vi "wheeltrackerGo_Stop8.6.vi"() -> ()   [LabVIEW 2013]
uses:
  pass_fail.ctl
  <vilib>/DAQmx/write.llb/DAQmx Write (Digital Bool 1Line 1Point).vi
  <vilib>/DAQmx/read.llb/DAQmx Read (Analog DBL 1Chan 1Samp).vi
  <vilib>/DAQmx/read.llb/DAQmx Read (Digital Bool 1Line 1Point).vi
  <vilib>/DAQmx/create/channels.llb/DAQmx Create Channel (DO-Digital Output).vi
  <vilib>/DAQmx/miscellaneous.llb/DAQmx Fill In Error Info.vi
  <vilib>/DAQmx/create/channels.llb/DAQmx Create Channel (DI-Digital Input).vi
  <vilib>/DAQmx/create/channels.llb/DAQmx Create Channel (AI-Voltage-Basic).vi
  <vilib>/Utility/file.llb/Write To Spreadsheet File (string).vi
  <vilib>/Utility/file.llb/Write To Spreadsheet File (DBL).vi
panel:
  out "Sample Time Interval (ms)":u32=20
  in  "Sample Rate (Hz)":u32=50 min=1 max=200
  out "Elapsed Time (s)":dbl
  out "x-y 2":dbl
  out "Time has Elapsed":bool
  in  "Time Before Delay End":dbl
  in  "Camera Trigger":tag="Dev2/port0/line3"
  in  "Lick Thr":dbl
  out "Ana Lick?":bool
  in  "x":dbl=1.0
  out "x*y":dbl
  in  "Scale":dbl=1.0 format="%#_13g"
  in  "Analog Lick Chan":tag="Dev2/ai0"
  out "Prev Stim?":bool
  in  "Alternate Stim?":bool
  in  "Thr Opto \nRun Factor":dbl=0.05
  out "Opto RUN Thr":bool
  in  "Opto Channel":tag="Dev2/port0/line4"
  in  "Opto Cond":T1(radio)=enum."Opto OFF"
  out "OptoON":bool
  in  "min speed":dbl=0.005
  in  "Stop Before Go?":bool
  in  "Fails 2 Penalty":dbl=3.0
  in  "Fails Penalty (s)":dbl=4.0
  out "Conseq. Fails":i32
  in  "control puff interval":dbl=1.0
  in  "control puff":bool
  in  "lick fail":bool
  out "NoGo & Stop":bool caption="Boolean"
  in  "NoGo Prob?":dbl
  out "NoGo?":bool
  in  "No-Go/Stop Channel":tag="Dev2/port0/line6"
  out "Success %":dbl
  in  "Buffer Time (s)":dbl
  in  "Stop Fail Repeat Prob 2":dbl caption="STOP\nRepeat Prob on fail"
  out "In":bool
  in  "Digital In Channel":tag="Dev2/port0/line5"
  out "Stop Speed Reached":bool
  out "Go/Stop?":bool
  out "Stop Flash # 2":dbl
  in  "Stop Stim On (s)":dbl=0.5 format="%#_13g"
  out "Stop Delay \nActual (s)":dbl
  in  "Delay Max (s)":dbl=4.0 format="%#_13g"
  in  "Delay Min (s)":dbl=2.0 format="%#_13g"
  out "Stop Thres Reached":bool
  in  "Stop Thres.":dbl=1.0 format="%#_13g"
  in  "Stop Flash #":dbl
  in  "Stim On (s)":dbl=0.1 format="%#_13g"
  out "Speed":dbl format="%#_13g"
  in  "Stop":bool
  in  "Stop Fail Speed":dbl=3.0
  out "Stop Slide":dbl(slide) max=2.0 scale=0.0..2.0
  in  "Stop Prob":dbl=0.5 caption="Probability" min=0.0 max=1.0 step=0.1 format="%.1f"
  in  "Stop Duration":dbl=2.0 caption="Stop Dur (s)"
  in  "Current Period":u8
  in  "Current Trial":u16
  in  "Fail sound play":bool
  in  "Pass sound play":bool
  in  "Fail Sound":string(combo)="C:\\Windows\\Media\\ringout.wav"
  in  "Pass Sound":string(combo)="C:\\Windows\\Media\\windows error.wav"
  in  "Fail Repeat Prob":dbl caption="GO\nRepeat Prob on fail"
  out "reset distance":bool
  out "give reward":bool
  in  "Shutter Click":bool
  out "Slide Trial #":u8(slide) max=5 scale=0.0..5.0
  out "Current Thres":dbl
  in  "exit":bool
  in  "Go/noGo Reward Thres":dbl=5.0 caption="Threshold"
  in  "Wheel Test":bool
  in  "Init Abort Threshold":dbl=6.0 caption="Abort Threshold"
  in  "Room light test":bool
  in  "Solid test":bool
  in  "Flash test":bool
  out "Go/No-go LED":bool
  in  "Room Light Channel":tag="Dev2/port0/line0"
  in  "Shutter Duration":dbl=0.05
  in  "Wheel Monitor Channel":refnum<visa-resource-name>="USB0::0x046D::0xC245::NI-VISA-0::RAW"
  in  "Number of Trials":u16=1
  out "Room light":bool
  out "Slide Inter-trail":dbl(slide) max=6.0 scale=-1.0..6.0
  out "Fail Delay Actual":dbl caption="Actual(s)"
  in  "Fail Delay Max":dbl=6.0 caption="Max(s)"
  in  "Fail Delay Min":dbl=6.0 caption="Min(s)"
  out "Pass Delay Actual":dbl caption="Actual(s)"
  in  "Pass Delay Max":dbl=3.0 caption="Max(s)"
  in  "Pass delay Min":dbl=3.0 caption="Min(s)"
  in  "Reward time (s)":dbl=2.0
  out "Slide Reward":dbl(slide) max=2.0 scale=0.0..2.0
  out "Slide go/no-go":dbl(slide) max=12.0 scale=0.0..12.0
  out "Slide Delay":dbl(slide) max=18.879 scale=0.0..18.879
  out "Thres reached":bool
  in  "Go Duration":dbl=12.0 caption="Go Dur (s)"
  out "Init Delay Actual":dbl caption="Actual(s)"
  in  "Init Delay Max":dbl=2.0 caption="Max(s)"
  in  "Init Delay Min(s)":dbl=1.0 caption="Min(s)"
  in  "Flashing Interval":dbl=0.1
  in  "Go Channel":tag="Dev2/port0/line1"
  in  "Data File Location":path
  in  "Queue":T2
  in  "Save":bool=TRUE
  in  "Log rate":dbl=0.01 min=0.0 max=1.0
  in  "Lin rate":dbl=0.01 min=0.0 max=1.0
  in  "Exp rate":dbl=0.01 min=0.0 max=1.0
  in  "Decay":enum32{"None", "Exp", "Lin", "Log"}(radio)
  in  "Wheel direction":bool=TRUE
  out "Shutter":bool
  in  "Run Trials":bool
  in  "Shutter Channel":tag="Dev2/port0/line2"
  out "Distance":dbl
  out "Reward Count":dbl
  out "Wheel Graph":cluster{dbl, dbl, i16, dbl, dbl}(graph)
  # "NOT USED"
  # "Initial Delay Period"
  # "Go/No-Go Period"
  # "Stop Period"
  # "Reward Period"
  # "Inter-trial Delay Period"
  # "Go-Stop Delay"
  # "Pass"
  # "Fail"
  # "*Update data saving parameters*"
  # "Decay rate"
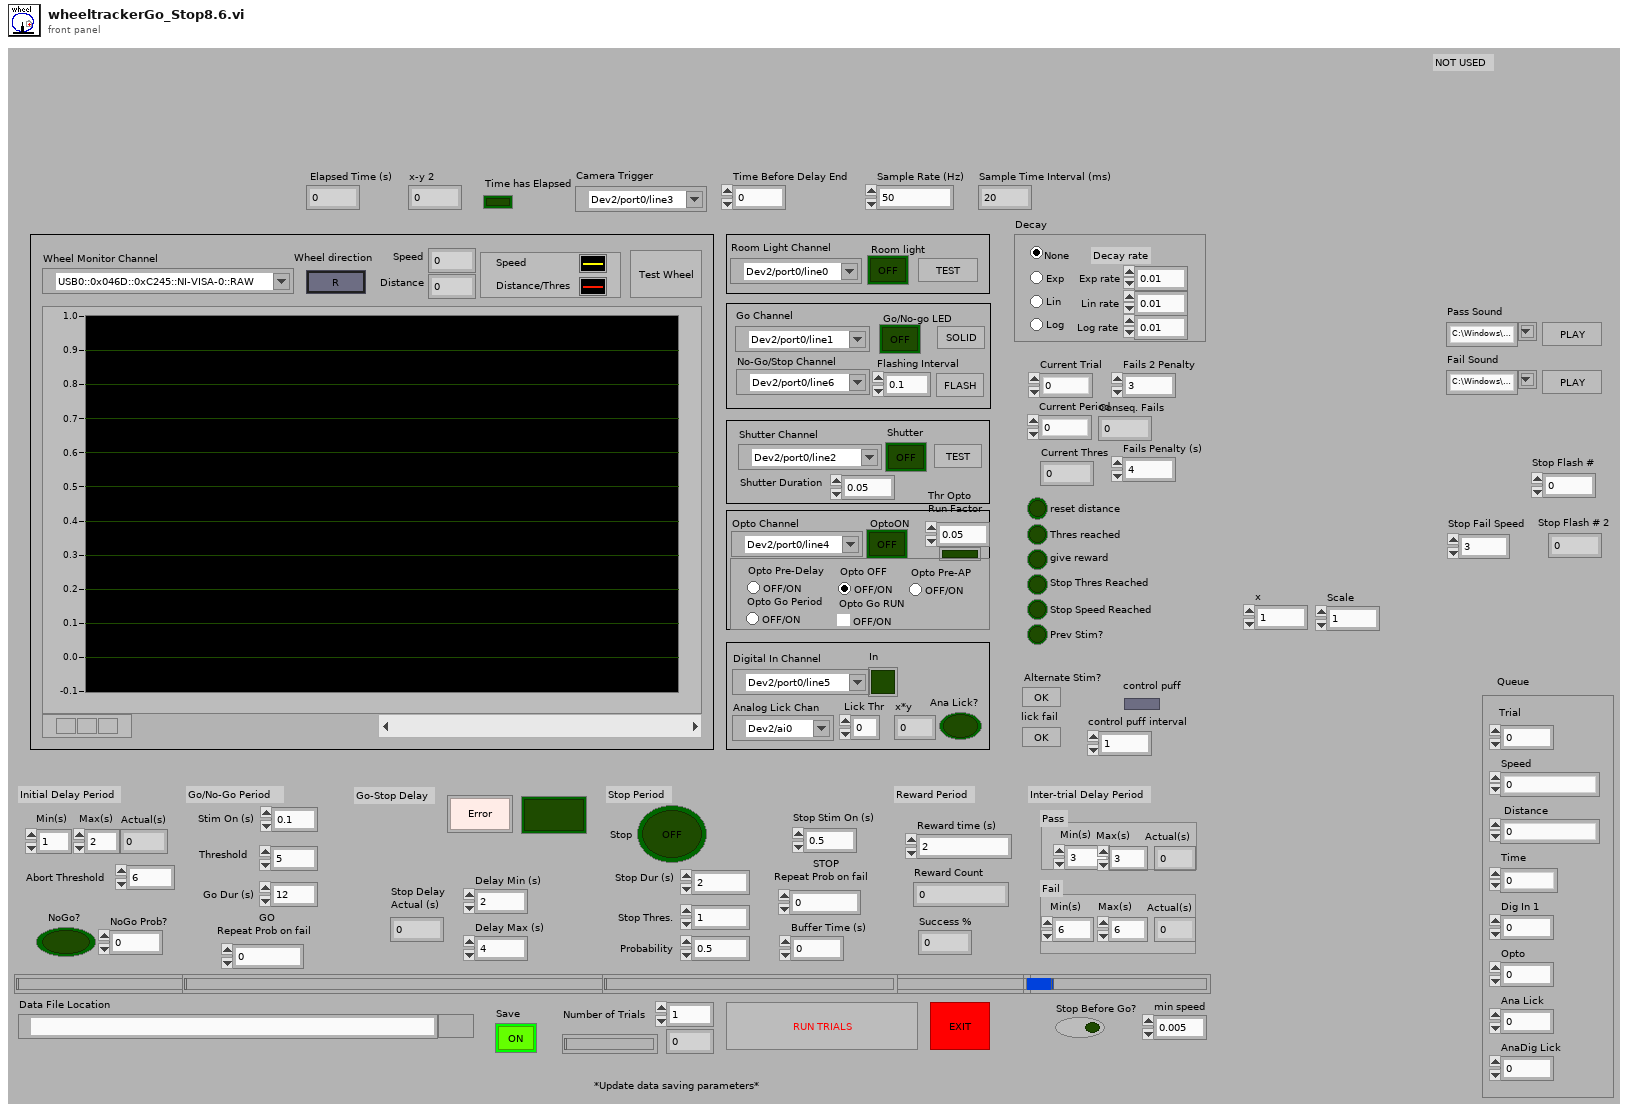
[diagram p1: front panel]
types:
  T1 = enum32{"Opto Pre-Delay", "Opto Go Period", "Opto OFF", "Opto Go RUN", "Opto Pre-AP"}
  T2 = cluster{"Trial":dbl, "Speed":dbl, " Distance":dbl, "Time":dbl, "Dig In 1":dbl, "Opto":dbl, "Ana Lick":dbl, "AnaDig Lick":dbl}
  T3 = enum16{"open", "replace", "create", "open or create", "replace or create", "replace or create with confirmation"}
  T4 = typedef "pass_fail.ctl" = enum32{"passed", "init fail", "go/no-go fail", "Stop Fail", "aborted"}
  T5 = cluster{"task out":refnum<k21>, "task out":refnum<k21>}
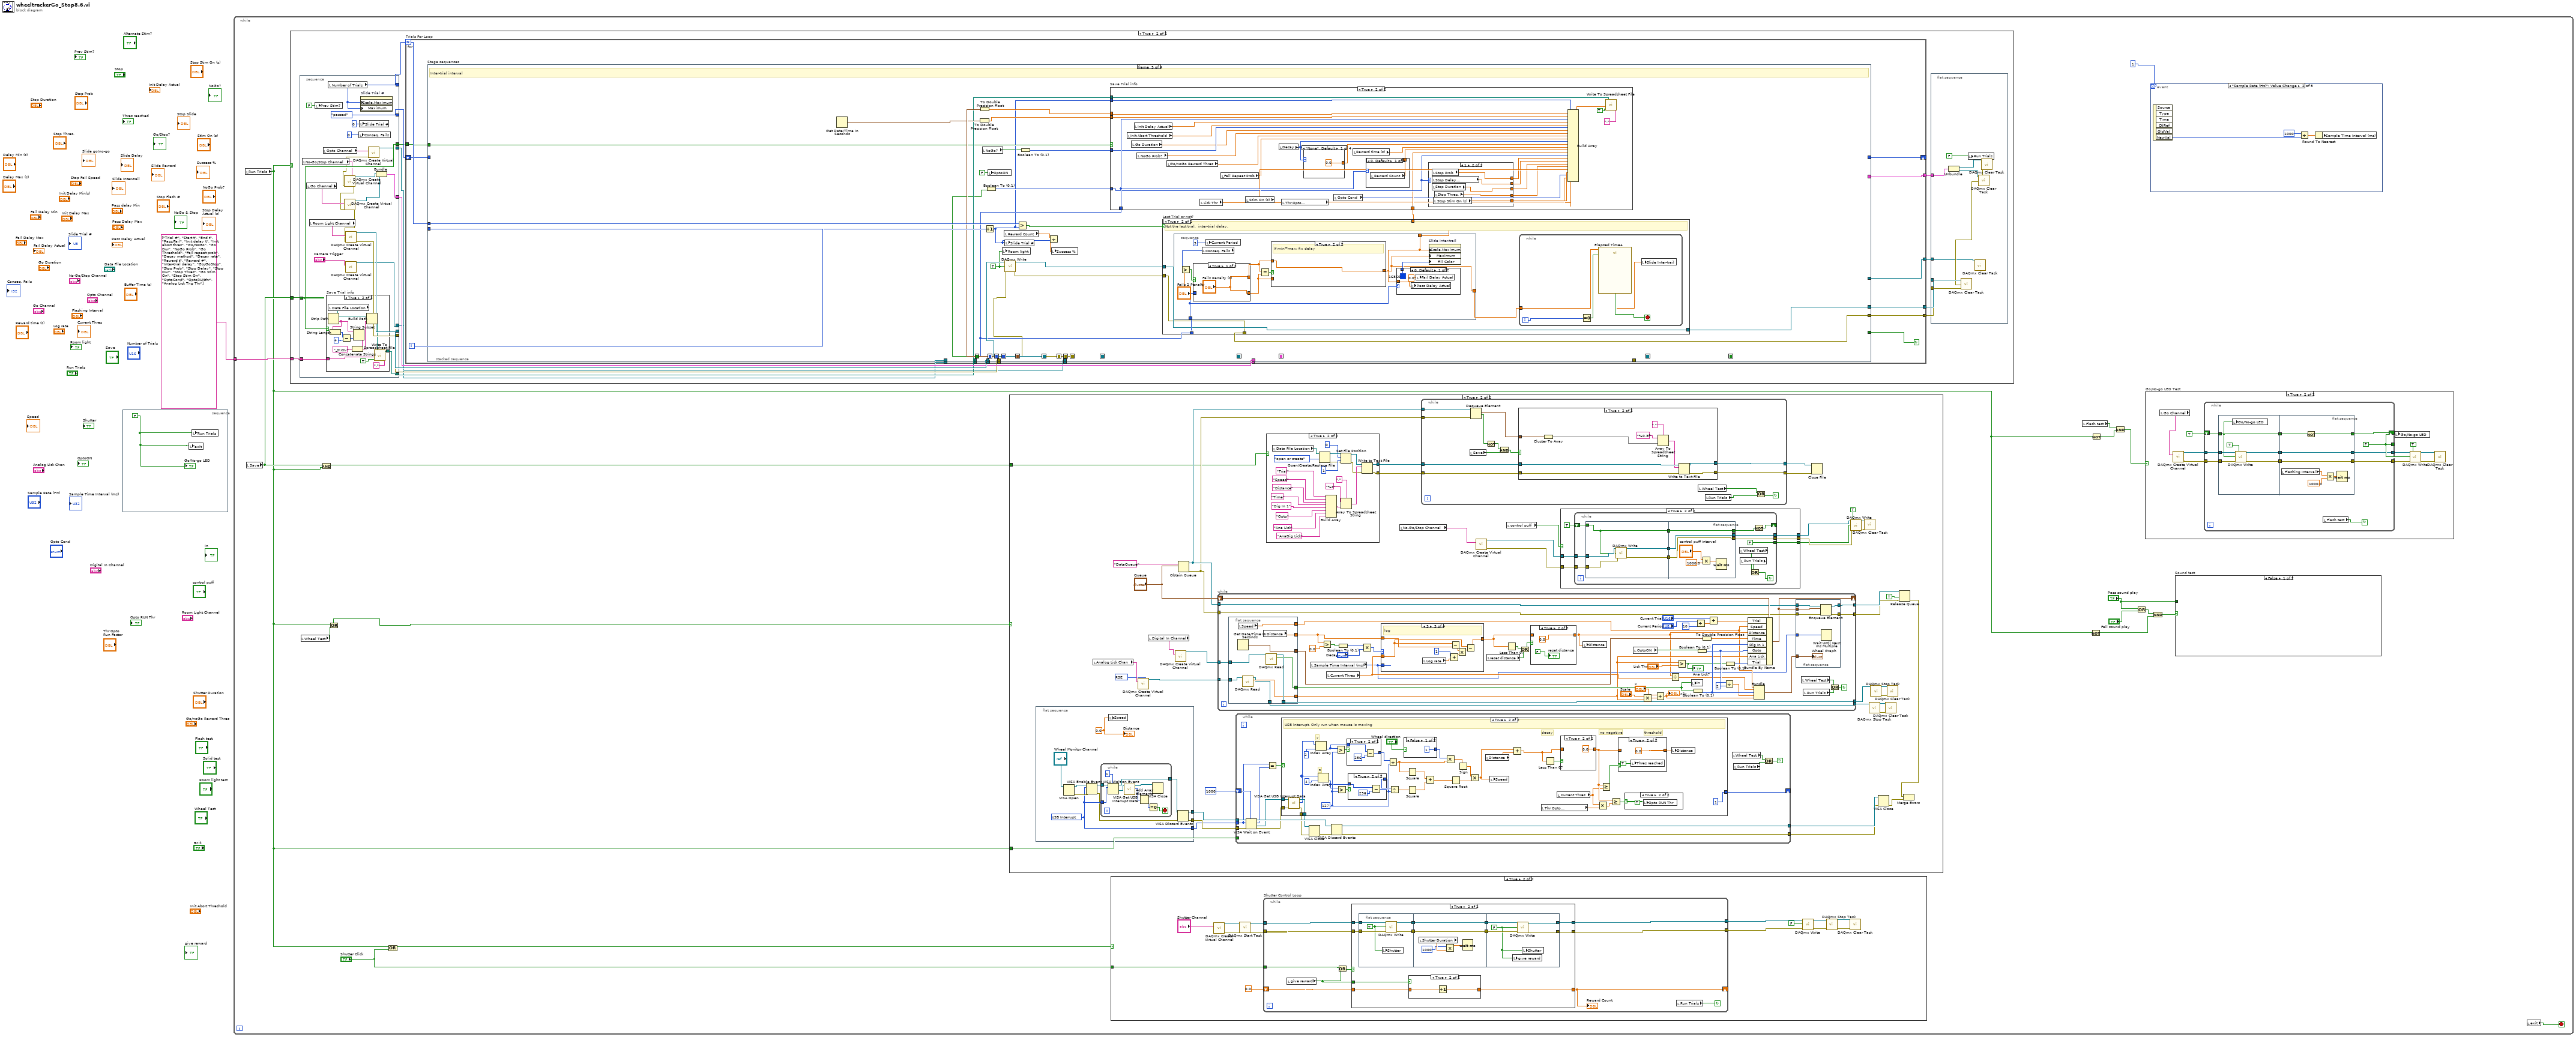
[diagram p0: block diagram]
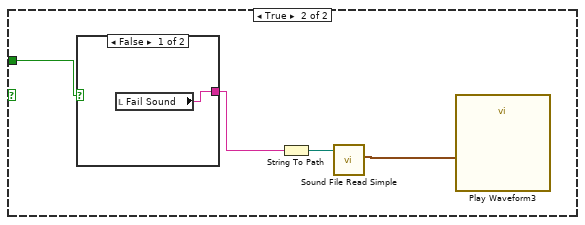
[diagram p3: hidden frame]
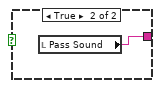
[diagram p4: hidden frame]
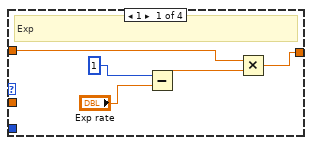
[diagram p10: hidden frame]
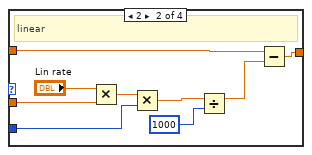
[diagram p11: hidden frame]
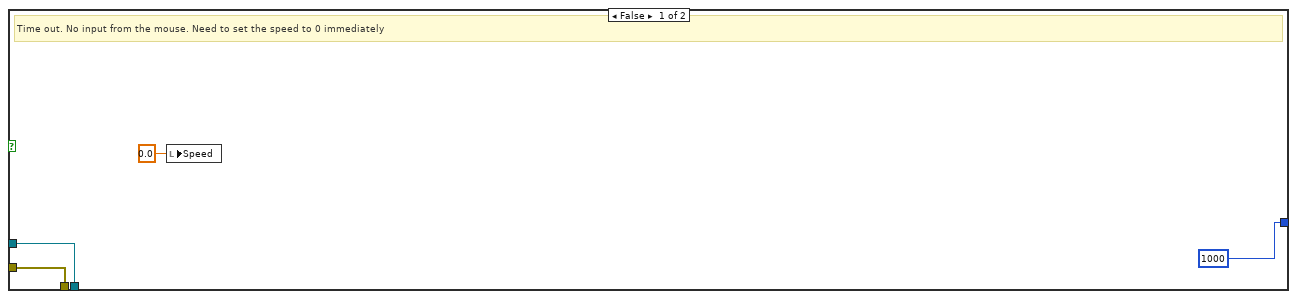
[diagram p13: hidden frame]
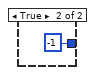
[diagram p17: hidden frame]
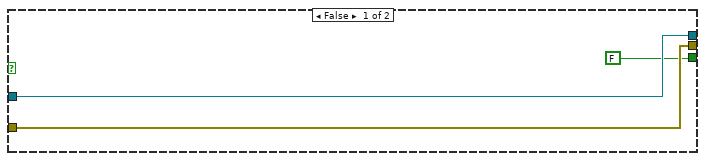
[diagram p20: hidden frame]
diagram:
  n1 = stacked-sequence {
    frame #0 {
      w2 = FALSE ("start")
      n2 = local write "exit"(w2) -> ()
      n3 = local write "Run Trials"(w2) -> ()
      "Go/No-go LED" <- w2
    }
  }
  n4 = while {
    tunnel: string[] ["Trial #", "Start t", "End t", "Pass/Fail", "Init delay t", "Init abort thres", "Go/NoGo", "Go Dur", "NoGo Prob", "Go Threshold", "Fail repeat prob", "Decay method", "Decay rate", "Reward t", "Reward #", "Inter-trial delay", "Go/GoStop", "Stop Prob", "Stop Delay", "Stop Dur", "Stop Thres", "Go Stim On", "Stop Stim On", "OptoCond", "OptoRUNthr", "Analog Lick Trig Thr"] -> [w8]
    stop <- w20 stop-if-true
    n5 = local read "Run Trials"() -> (w5:bool)
    n6 = local read "Save"() -> (w7:bool)
    n7 = case shown="True" w5 {
      tunnel: w8 -> [_ w464]
      tunnel: w7 -> [_ w463]
      frame False {
      }
      frame True {
        n8 = stacked-sequence {
          tunnel: [w505] -> w473
          tunnel: [w502] -> w472
          tunnel: [w490] -> w471
          tunnel: [w500] -> w468
          tunnel: [pass_fail."passed" ("How it ended")] -> w466
          tunnel: [w498] -> w465
          tunnel: w464 -> [w497]
          tunnel: w463 -> [w496]
          tunnel: [w496] -> w462
          tunnel: [w487] -> w461
          tunnel: [w483] -> w460
          frame #0 {
            n9 = local read "No-Go/Stop Channel"() -> (w493:tag)
            n10 = local read "Go Channel"() -> (w495:tag)
            n11 = local read "Room Light Channel"() -> (w503:tag)
            n12 = local write "Prev Stim?"(FALSE ("Prev Stim?")) -> ()
            n13 = local read "Opto Channel"() -> (w488:tag)
            n14 = case "Save Trial info" shown="True" w496 {
              tunnel: [_ w509] -> w498
              tunnel: w497 -> [_ w508]
              frame False {
              }
              frame True {
                n15 = local read "Data File Location"() -> (w519:path)
                n16 = Strip Path(path=w519) -> (stripped path=w512:path, name=w518:string)
                n17 = String Length(string=w518) -> (length=w516:i32)
                n18 = Subtract(x=w516, y=4) -> (x-y=w510:i32)
                n19 = String Subset(string=w518, length (rest)=w510) -> (substring=w515:string)  [unwired: 1 in]
                n20 = Concatenate Strings(w515, "_tr.csv") -> (w513:string)
                n21 = Build Path(base path=w512, name or relative path=w513) -> (appended path=w511:path)
                n22 = call-poly <vilib>:"Write To Spreadsheet File.vi"("delimiter (\\t)"="," ("delimiter (\\t)"), "append to file? (new file:F)"=TRUE, "1D data"=w508, "file path (dialog if empty)"=w511) -> ("new file path (Not A Path if cancelled)"=w509:path)  [unwired: 4 in]
              }
            }
            n23 = local read "Number of Trials"() -> (w505:u16)
            n24 = call-poly <vilib>:"DAQmx Create Virtual Channel.vi"("lines"="Camera Trigger") -> ("task out"=w483:refnum<k21>)  [unwired: 13 in, 1 out]
            n25 = local write "Conseq. Fails"(u8 0 ("Slide Trial #")) -> ()
            n26 = local write "Slide Trial #"(u8 0 ("Slide Trial #")) -> ()
            n27 = property on="Slide Trial #" class="Slide (strict)"("Scale.Maximum"=w505, "Maximum"=w505) -> ()  [unwired: 2 in, 2 out]
            n28 = call-poly <vilib>:"DAQmx Create Virtual Channel.vi"("lines"=w488) -> ("task out"=w487:refnum<k21>, "error out"=w486:errorcluster)  [unwired: 13 in]
            n29 = call-poly <vilib>:"DAQmx Create Virtual Channel.vi"("lines"=w493, "error in"=w486) -> ("task out"=w491:refnum<k21>, "error out"=w494:errorcluster)  [unwired: 12 in]
            n30 = call-poly <vilib>:"DAQmx Create Virtual Channel.vi"("lines"=w495, "error in"=w494) -> ("task out"=w492:refnum<k21>, "error out"=w501:errorcluster)  [unwired: 12 in]
            n31 = call-poly <vilib>:"DAQmx Create Virtual Channel.vi"("lines"=w503, "error in"=w501) -> ("task out"=w502:refnum<k21>, "error out"=w500:errorcluster)  [unwired: 12 in]
            n32 = Bundle("task out"=w491, "task out"=w492) -> (w490:T5)  [unwired: 1 in]
          }
        }
        n33 = for "Trials For Loop" {
          N: w473 -> [w534]
          tunnel: w472 -> [w533]
          tunnel: w471 -> [w532]
          tunnel: [w523] -> w470
          tunnel: [w531] -> w469
          tunnel: w468 -> [w530]
          tunnel: [w529] -> w467
          shift-right: [w526] -> _
          shift-left: w466 -> [w527]
          tunnel: w465 -> [w525]
          tunnel: w462 -> [w524]
          tunnel: w461 -> [w522]
          tunnel: w460 -> [w521]
          tunnel: [w520] -> w459
          i -> [w535]
          stop <- w528 continue-if-true
          # "Repeat Trials  For loop."
          n34 = stacked-sequence "Stage sequences" {
            seq-local: [w563 _ _ _ _ _] -> [_ w678 _ _ _ _]
            seq-local: [_ _ w858 _ _ _] -> [_ _ _ w920 w957 _]
            seq-local: [w561 _ _ _ _ _] -> [_ _ _ _ w965 _]
            seq-local: [w549 _ _ _ _ _] -> [_ w676 _ _ _ _]
            seq-local: [_ w675 _ _ _ _] -> [_ _ w857 _ _ _]
            seq-local: [w550 _ _ _ _ _] -> [_ _ _ _ w963 _]
            seq-local: [_ w673 _ _ _ _] -> [_ _ w852 _ _ _]
            seq-local: [_ w671 _ _ _ _] -> [_ _ w853 _ _ _]
            seq-local: [_ _ w856 _ _ _] -> [_ _ _ _ w955 _]
            seq-local: [_ w672 _ _ _ _] -> [_ _ w854 _ _ _]
            seq-local: [_ _ w852 _ _ _] -> [_ _ _ _ w950 _]
            seq-local: [w548 _ _ _ _ _] -> [_ w670 _ _ _ _]
            seq-local: [_ w669 _ _ _ _] -> [_ _ _ _ _ _]
            seq-local: [w538 _ _ _ _ _] -> [_ _ w851 _ _ _]
            tunnel: w535 -> [w546 w668 _ _ w968 _]
            tunnel: w534 -> [_ _ _ _ w967 _]
            tunnel: w533 -> [w562 _ _ _ _ _]
            tunnel: w532 -> [_ w677 _ _ _ _]
            tunnel: [_ _ _ _ w953 _] -> w531
            tunnel: w530 -> [w560 _ _ _ _ _]
            tunnel: [_ _ _ _ w951 _] -> w529
            tunnel: [_ _ _ _ _ w1068] -> w528
            tunnel: w527 -> [_ w674 _ _ _ _]
            tunnel: [_ _ _ w920 _ _] -> w526
            tunnel: w525 -> [_ _ _ _ w959 _]
            tunnel: w524 -> [_ _ _ _ w956 _]
            tunnel: [_ _ w855 _ _ _] -> w523
            tunnel: w522 -> [w555 _ _ _ _ _]
            tunnel: w521 -> [w545 _ _ _ _ _]
            tunnel: [w536 _ _ _ _ _] -> _
            tunnel: [_ _ w851 _ _ _] -> w520
            frame #0 {
              w547 = FALSE ("data")
              # "Fix/Random Initial Delay"
              n35 = flat-sequence {
                tunnel: w562 -> [w587]
                tunnel: [w586] -> w561
                tunnel: w560 -> [w585]
                tunnel: [w584] -> w551
                tunnel: [w581] -> w550
                tunnel: w546 -> [w580]
                tunnel: [w588] -> w559
                tunnel: [w603] -> w564
                tunnel: w559 -> [w603]
                frame #0 {
                  w574 = FALSE
                  w583 = FALSE ("data")
                  w577 = 0.0
                  n36 = Increment(x=w580) -> (x+1=w579:i32)
                  n37 = Get Date/Time In Seconds() -> (seconds since 1Jan1904=w581:timestamp)
                  n38 = local write "Current Trial"(w579) -> ()
                  n39 = local write "Current Period"(1) -> ()
                  n40 = local write "Stop Thres Reached"(w574) -> ()
                  n41 = local write "Thres reached"(w574) -> ()
                  n42 = local write "reset distance"(TRUE) -> ()
                  n43 = local write "give reward"(w574) -> ()
                  n44 = local write "OptoON"(w574) -> ()
                  n45 = local read "Init Delay Min(s)"() -> (w575:dbl)
                  n46 = local read "Init Delay Max"() -> (w582:dbl)
                  n47 = local write "Room light"(w583) -> ()
                  n48 = call-poly <vilib>:"DAQmx Write.vi"("task/channels in"=w587, "data"=w583, "error in"=w585) -> ("task out"=w586:refnum<k21>, "error out"=w584:errorcluster)  [unwired: 10 in, 1 out]
                  n49 = Equal?(x=w582, y=w575) -> (x = y?=w589:bool)
                  n50 = case shown="False" w589 {
                    tunnel: [w595 w602] -> w588
                    tunnel: w582 -> [w594 _]
                    tunnel: w575 -> [w593 _]
                    frame False {
                      # "If min != max; random delay betwen min and max"
                      n51 = Subtract(x=w594, y=w593) -> (x-y=w592:dbl)
                      n52 = Random Number (0-1)() -> (number: 0 to 1=w591:dbl)
                      n53 = Multiply(x=w591, y=w592) -> (x*y=w601:dbl)
                      n54 = Add(x=w601, y=w593) -> (x+y=w600:dbl)
                      n55 = Multiply(x=w600, y=1000) -> (x*y=w597:dbl)
                      n56 = Round To Nearest(number=w597) -> (nearest integer value=w596:dbl)
                      n57 = Divide(x=w596, y=1000) -> (x/y=w595:dbl)
                    }
                    frame True {
                      # "If min=max; fix delay"
                      n58 = local read "Init Delay Min(s)"() -> (w602:dbl)
                    }
                  }
                  n59 = local write "Slide Inter-trail"(w577) -> ()
                  n60 = local write "Slide Reward"(w577) -> ()
                  n61 = local write "Slide Delay"(w577) -> ()
                  n62 = local write "Slide go/no-go"(w577) -> ()
                  n63 = local write "Stop Slide"(w577) -> ()
                  n64 = local read "Init Abort Threshold"() -> (w590:dbl)
                  n65 = local write "Current Thres"(w590) -> ()
                  n66 = local write "Init Delay Actual"(w588) -> ()
                  n67 = property on="Slide Delay" class="Slide (strict)"("Scale.Maximum"=w588, "Maximum"=w588) -> ()  [unwired: 2 in, 2 out]
                }
                frame #1 {
                  n68 = while {
                    i -> [w606]
                    stop <- w607 stop-if-true
                    n69 = Equal To 0?(x=w606) -> (x = 0?=w605:bool)
                    n70 = call "Elapsed Time9"("Time Target (s)"=2.0, "Reset"=w605) -> ("Time has Elapsed"=w607:bool)  [unwired: 10 in, 7 out]
                  }
                }
              }
              n71 = call <vilib>:"DAQmx Start Task.vi"("task/channels in"=w545) -> ("task out"=w544:refnum<k21>, "error out"=w543:errorcluster)  [unwired: 13 in]
              n72 = call <vilib>:"DAQmx Start Task.vi"("task/channels in"=w555, "error in"=w551) -> ("task out"=w556:refnum<k21>, "error out"=w554:errorcluster)  [unwired: 12 in]
              n73 = while {
                tunnel: w564 -> [w615]
                tunnel: [w637] -> w565
                tunnel: w556 -> [w632]
                tunnel: [w631] -> w558
                tunnel: w554 -> [w629]
                tunnel: [w628] -> w553
                tunnel: w546 -> [w621]
                tunnel: w544 -> [w617]
                tunnel: w543 -> [w616]
                tunnel: [w609] -> w542
                tunnel: [w610] -> w541
                i -> [w640]
                stop <- w636 stop-if-true
                # "delay time loop"
                n74 = Subtract(x=w615, y="Time Before Delay End") -> (x-y=w613:dbl)
                "x-y 2" <- w613
                n75 = local read "Alternate Stim?"() -> (w618:bool)
                n76 = local read "Opto Cond"() -> (w630:T1)
                n77 = Quotient & Remainder(x=w621, y=2) -> (x-y*floor(x/y)=w620:i32)  [unwired: 1 out]
                n78 = Equal To 0?(x=w620) -> (x = 0?=w619:bool)
                n79 = local read "Thres reached"() -> (w634:bool)
                n80 = Equal To 0?(x=w640) -> (x = 0?=w611:bool)
                n81 = call "Elapsed Time11"("Time Target (s)"=w613, "Reset"=w611) -> ("Elapsed Time (s)"=→"Elapsed Time (s)":dbl, "Time has Elapsed"=w612:bool)  [unwired: 10 in, 6 out]
                "Time has Elapsed" <- w612
                n82 = call-poly <vilib>:"DAQmx Write.vi"("task/channels in"=w617, "data"=w612, "error in"=w616) -> ("task out"=w609:refnum<k21>, "error out"=w610:errorcluster)  [unwired: 10 in, 1 out]
                n83 = local read "Speed"() -> (w638:dbl)
                n84 = call "Elapsed Time"("Time Target (s)"=w615, "Reset"=w611) -> ("Elapsed Time (s)"=w626:dbl, "Time has Elapsed"=w635:bool)  [unwired: 10 in, 6 out]
                n85 = Subtract(x=w615, y=w626) -> (x-y=w625:dbl)
                n86 = Less?(x=w625, y=1.0) -> (x < y?=w623:bool)
                n87 = case shown="False" w618 {
                  tunnel: w630 -> [w643 w652]
                  tunnel: [w642 w651] -> w627
                  tunnel: w623 -> [w641 w650]
                  tunnel: w619 -> [_ w649]
                  frame False {
                    n88 = case shown="\"Opto Pre-AP\"" w643 {
                      tunnel: [TRUE FALSE FALSE FALSE w648] -> w642
                      tunnel: w641 -> [_ _ _ _ w648]
                      frame "Opto Pre-Delay", Default {
                      }
                      frame "Opto Go Period" {
                      }
                      frame "Opto OFF" {
                      }
                      frame "Opto Go RUN" {
                      }
                      frame "Opto Pre-AP" {
                      }
                    }
                  }
                  frame True {
                    n89 = case shown="True" w649 {
                      tunnel: w652 -> [_ w656]
                      tunnel: [FALSE w655] -> w651
                      tunnel: w650 -> [_ w654]
                      frame True {
                      }
                      frame False {
                        n90 = case shown="\"Opto Pre-AP\"" w656 {
                          tunnel: [FALSE TRUE FALSE FALSE w661] -> w655
                          tunnel: w654 -> [_ _ _ _ w661]
                          frame "Opto OFF", Default {
                          }
                          frame "Opto Pre-Delay" {
                          }
                          frame "Opto Go Period" {
                          }
                          frame "Opto Go RUN" {
                          }
                          frame "Opto Pre-AP" {
                          }
                        }
                      }
                    }
                  }
                }
                n91 = local write "OptoON"(w627) -> ()
                n92 = call-poly <vilib>:"DAQmx Write.vi"("task/channels in"=w632, "data"=w627, "error in"=w629) -> ("task out"=w631:refnum<k21>, "error out"=w628:errorcluster)  [unwired: 10 in, 1 out]
                n93 = case shown="False" "Stop Before Go?" {
                  tunnel: w638 -> [_ w667]
                  tunnel: [w663 w665] -> w637
                  tunnel: w635 -> [w663 _]
                  tunnel: w634 -> [w662 _]
                  tunnel: [w662 FALSE ("y")] -> w633
                  frame False {
                  }
                  frame True {
                    n94 = Less?(x=w667, y="min speed") -> (x < y?=w665:bool)
                  }
                }
                n95 = local write "Slide Delay"(w626) -> ()
                n96 = Or(x=w637, y=w633) -> (x .or. y?=w636:bool)
              }
              n97 = call-poly <vilib>:"DAQmx Write.vi"("task/channels in"=w542, "data"=FALSE, "error in"=w541) -> ("task out"=w539:refnum<k21>, "error out"=w537:errorcluster)  [unwired: 10 in, 1 out]
              n98 = call-poly <vilib>:"DAQmx Write.vi"("task/channels in"=w558, "data"=w547, "error in"=w553) -> ("task out"=w557:refnum<k21>, "error out"=w552:errorcluster)  [unwired: 10 in, 1 out]
              n99 = local write "OptoON"(w547) -> ()
              n100 = call <vilib>:"DAQmx Stop Task.vi"("task/channels in"=w539, "error in"=w537) -> ("task out"=w538:refnum<k21>, "error out"=w536:errorcluster)  [unwired: 12 in]
              n101 = call <vilib>:"DAQmx Stop Task.vi"("task/channels in"=w557, "error in"=w552) -> ("task out"=w548:refnum<k21>, "error out"=w549:errorcluster)  [unwired: 12 in]
              n102 = flat-sequence {
                tunnel: w565 -> [w567]
                tunnel: [w566] -> w563
                frame #0 {
                  n103 = case shown="True" w567 {
                    tunnel: [pass_fail."init fail" ("How it ended") pass_fail."passed" ("How it ended")] -> w566
                    frame False {
                      # "see if this period passed or failed"
                    }
                    frame True {
                    }
                  }
                }
                frame #1 {
                  n104 = local write "reset distance"(TRUE) -> ()
                  n105 = local write "Thres reached"(FALSE) -> ()
                  n106 = local write "Opto RUN Thr"(FALSE ("Opto RUN Thr")) -> ()
                  n107 = Wait (ms)(milliseconds to wait=u32 50) -> ()  [unwired: 1 out]
                }
              }
            }
            frame #1 {
              # "Go/No-go Period"
              n108 = stacked-sequence {
                frame #0 {
                  n109 = local read "Go/noGo Reward Thres"() -> (w680:dbl)
                  n110 = local write "Current Period"(2) -> ()
                  n111 = local write "Current Thres"(w680) -> ()
                }
              }
              n112 = case shown="\"passed\", Default" w678 {
                selector: w678 -> [_ w850]
                tunnel: [w710 w850] -> w671
                tunnel: w677 -> [w701 w849]
                tunnel: [w698 w849] -> w672
                tunnel: w676 -> [w709 w848]
                tunnel: [w687 w848] -> w675
                tunnel: w674 -> [w705 _]
                tunnel: [w703 w847] -> w673
                tunnel: w670 -> [w692 w846]
                tunnel: [w684 w846] -> w669
                tunnel: w668 -> [w682 _]
                frame "passed", Default {
                  (unwired) enum32{"passed", "failed", "aborted"}."failed" ("How it ended")
                  n113 = flat-sequence {
                    tunnel: w705 -> [w740]
                    tunnel: [w741] -> w696
                    tunnel: [w731] -> w695
                    tunnel: [w777] -> w703
                    tunnel: [w778] -> w711
                    tunnel: w696 -> [w778]
                    tunnel: w695 -> [w777]
                    frame #0 {
                      n114 = local read "NoGo Prob?"() -> (w735:dbl)
                      n115 = Random Number (0-1)() -> (number: 0 to 1=w738:dbl)
                      n116 = Greater?(x=w735, y=w738) -> (0:w737:bool)
                      n117 = Greater?(x=w735, y=0.0) -> (0:w733:bool)
                      n118 = local write "NoGo?"(w737) -> ()
                      n119 = Random Number (0-1)() -> (number: 0 to 1=w743:dbl)
                      n120 = local read "Stop Prob"() -> (w744:dbl)
                      n121 = Greater?(x=w744, y=w743) -> (0:w742:bool)
                      n122 = case "pass or fail?" shown="0, Default" w740 {
                        tunnel: w742 -> [w762 w765 w772]
                        tunnel: [w762 w764 w771] -> w739
                        frame 0, Default {
                          # "no repeat"
                        }
                        frame 1, 2 {
                          n123 = Random Number (0-1)() -> (number: 0 to 1=w767:dbl)
                          n124 = Less?(x=w767, y="Fail Repeat Prob") -> (x < y?=w763:bool)
                          n125 = case "repeat?" shown="True" w763 {
                            tunnel: w765 -> [w768 _]
                            tunnel: [w768 w769] -> w764
                            tunnel: w763 -> [_ w769]
                            frame False {
                              # "no repeat"
                            }
                            frame True {
                              # "repeat"
                            }
                          }
                        }
                        frame 3 {
                          n126 = Random Number (0-1)() -> (number: 0 to 1=w774:dbl)
                          n127 = Less?(x=w774, y="Stop Fail Repeat Prob 2") -> (x < y?=w770:bool)
                          n128 = case shown="False" w770 {
                            tunnel: [w775 w776] -> w771
                            tunnel: w772 -> [w775 _]
                            tunnel: w770 -> [_ w776]
                            frame False {
                            }
                            frame True {
                            }
                          }
                        }
                      }
                      n129 = local read "Stop"() -> (w736:bool)
                      n130 = And(x=w739, y=w736) -> (x .and. y?=w731:bool)
                      n131 = case shown="True" w731 {
                        tunnel: [w745 w761] -> w741
                        frame True {
                          n132 = local read "Delay Max (s)"() -> (w747:dbl)
                          n133 = local read "Delay Min (s)"() -> (w746:dbl)
                          n134 = Equal?(x=w746, y=w747) -> (x = y?=w748:bool)
                          n135 = case shown="False" w748 {
                            tunnel: w747 -> [_ w752]
                            tunnel: w746 -> [w749 w751]
                            tunnel: [w749 w750] -> w745
                            frame True {
                            }
                            frame False {
                              n136 = Random Number (0-1)() -> (number: 0 to 1=w759:dbl)
                              n137 = Subtract(x=w752, y=w751) -> (x-y=w760:dbl)
                              n138 = Multiply(x=w760, y=w759) -> (x*y=w758:dbl)
                              n139 = Add(x=w758, y=w751) -> (x+y=w757:dbl)
                              n140 = Multiply(x=w757, y=1000) -> (x*y=w754:dbl)
                              n141 = Round To Nearest(number=w754) -> (nearest integer value=w753:dbl)
                              n142 = Divide(x=w753, y=1000) -> (x/y=w750:dbl)
                            }
                          }
                          n143 = local write "Stop Delay \nActual (s)"(w745) -> ()
                        }
                        frame False {
                          n144 = local read "Go Duration"() -> (w761:dbl)
                        }
                      }
                      n145 = And(x=w733, y=w736) -> (x .and. y?=w732:bool)
                      n146 = local write "NoGo & Stop"(w732) -> ()
                      n147 = local write "Go/Stop?"(w731) -> ()
                      n148 = property on="Slide go/no-go" class="Slide (strict)"("Scale.Maximum"=w741, "Maximum"=w741) -> ()  [unwired: 2 in, 2 out]
                    }
                    frame #1 {
                      n149 = while {
                        i -> [w781]
                        stop <- w779 stop-if-true
                        n150 = Equal To 0?(x=w781) -> (x = 0?=w780:bool)
                        n151 = call "Elapsed Time10"("Time Target (s)"=0.0, "Reset"=w780) -> ("Time has Elapsed"=w779:bool)  [unwired: 10 in, 7 out]
                      }
                    }
                  }
                  n152 = local read "NoGo?"() -> (w681:bool)
                  n153 = local read "Opto Cond"() -> (w693:T1)
                  n154 = case shown="True" w681 {
                    tunnel: w701 -> [w725 w728]
                    tunnel: [w724 w727] -> w700
                    tunnel: [w723 w726] -> w697
                    frame True {
                      n155 = Unbundle(w725) -> ("task out"=w724:refnum<k21>, "task out"=w723:refnum<k21>)
                    }
                    frame False {
                      n156 = Unbundle(w728) -> ("task out"=w726:refnum<k21>, "task out"=w727:refnum<k21>)
                    }
                  }
                  n157 = call <vilib>:"DAQmx Start Task.vi"("task/channels in"=w700, "error in"=w709) -> ("task out"=w716:refnum<k21>, "error out"=w691:errorcluster)  [unwired: 12 in]
                  n158 = call <vilib>:"DAQmx Start Task.vi"("task/channels in"=w692, "error in"=w691) -> ("task out"=w694:refnum<k21>, "error out"=w690:errorcluster)  [unwired: 12 in]
                  n159 = while "LED loop" {
                    tunnel: w716 -> [w814]
                    tunnel: w690 -> [w813]
                    tunnel: [w812] -> w713
                    tunnel: [w795] -> w712
                    shift-right: [w811] -> w706
                    shift-left: TRUE -> [w809]
                    tunnel: w711 -> [w810]
                    tunnel: [w803] -> w702
                    tunnel: w694 -> [w797]
                    tunnel: w693 -> [w788]
                    tunnel: [w794] -> w686
                    tunnel: w682 -> [w790]
                    i -> [w791]
                    stop <- w801 stop-if-true
                    n160 = local read "Alternate Stim?"() -> (w792:bool)
                    n161 = Equal To 0?(x=w791) -> (x = 0?=w808:bool)
                    n162 = local read "NoGo?"() -> (w804:bool)
                    n163 = Quotient & Remainder(x=w790, y=2) -> (x-y*floor(x/y)=w787:i32)  [unwired: 1 out]
                    n164 = Equal To 0?(x=w787) -> (x = 0?=w786:bool)
                    n165 = local write "Go/No-go LED"(w809) -> ()
                    n166 = call "Elapsed Time2"("Time Target (s)"=w810, "Reset"=w808) -> ("Elapsed Time (s)"=w785:dbl, "Time has Elapsed"=w802:bool)  [unwired: 10 in, 6 out]
                    n167 = case shown="False" w804 {
                      tunnel: [w844 w845] -> w805
                      frame True {
                        n168 = local read "Stop Stim On (s)"() -> (w844:dbl)
                      }
                      frame False {
                        n169 = local read "Stim On (s)"() -> (w845:dbl)
                      }
                    }
                    n170 = call-poly <vilib>:"DAQmx Write.vi"("task/channels in"=w814, "data"=w809, "error in"=w813) -> ("task out"=w812:refnum<k21>, "error out"=w796:errorcluster)  [unwired: 10 in, 1 out]
                    n171 = local write "Slide go/no-go"(w785) -> ()
                    n172 = call "Elapsed Time6"("Time Target (s)"=w805, "Reset"=w808) -> ("Time has Elapsed"=w807:bool)  [unwired: 10 in, 7 out]
                    n173 = Less?(x=w785, y=1.0) -> (x < y?=w783:bool)
                    n174 = case shown="True" w792 {
                      tunnel: w788 -> [w817 w826]
                      tunnel: [w816 w825] -> w793
                      tunnel: w786 -> [_ w824]
                      tunnel: w783 -> [w815 w823]
                      frame False {
                        n175 = case shown="\"Opto Pre-AP\"" w817 {
                          tunnel: [FALSE w819 TRUE FALSE w822] -> w816
                          tunnel: w815 -> [_ w819 _ _ _]
                          frame "Opto Pre-Delay" {
                          }
                          frame "Opto Pre-AP" {
                          }
                          frame "Opto Go Period" {
                          }
                          frame "Opto OFF", Default {
                          }
                          frame "Opto Go RUN" {
                            n176 = local read "Opto RUN Thr"() -> (w822:bool)
                          }
                        }
                      }
                      frame True {
                        n177 = case shown="True" w824 {
                          tunnel: w826 -> [_ w830]
                          tunnel: [FALSE w829] -> w825
                          tunnel: w823 -> [_ w828]
                          frame True {
                          }
                          frame False {
                            n178 = case shown="\"Opto Pre-AP\"" w830 {
                              tunnel: [FALSE FALSE TRUE w834 w835] -> w829
                              tunnel: w828 -> [_ _ _ _ w835]
                              frame "Opto OFF", Default {
                              }
                              frame "Opto Pre-Delay" {
                              }
                              frame "Opto Go Period" {
                              }
                              frame "Opto Go RUN" {
                                n179 = local read "Opto RUN Thr"() -> (w834:bool)
                              }
                              frame "Opto Pre-AP" {
                              }
                            }
                          }
                        }
                      }
                    }
                    n180 = local write "OptoON"(w793) -> ()
                    n181 = call-poly <vilib>:"DAQmx Write.vi"("task/channels in"=w797, "data"=w793, "error in"=w796) -> ("task out"=w794:refnum<k21>, "error out"=w795:errorcluster)  [unwired: 10 in, 1 out]
                    n182 = Not And(1:w807, 2:TRUE) -> (0:w811:bool)
                    n183 = case shown="True" w804 {
                      tunnel: [w839 w842] -> w803
                      tunnel: w802 -> [w840 w841]
                      tunnel: [w838 w841] -> w799
                      frame False {
                        n184 = local read "Thres reached"() -> (w839:bool)
                        n185 = Or(x=w840, y=w839) -> (x .or. y?=w838:bool)
                      }
                      frame True {
                        n186 = local read "Thres reached"() -> (w843:bool)
                        n187 = Not(x=w843) -> (.not. x?=w842:bool)
                      }
                    }
                    n188 = case shown="False" "lick fail" {
                      tunnel: [FALSE w837] -> w800
                      frame False {
                      }
                      frame True {
                        n189 = local read "In"() -> (w837:bool)
                      }
                    }
                    n190 = Or(x=w800, y=w799) -> (x .or. y?=w801:bool)
                  }
                  n191 = And(x=FALSE, y=w706) -> (x .and. y?=w708:bool)
                  n192 = case "Pass or Fail" shown="False" w702 {
                    tunnel: [pass_fail."go/no-go fail" ("How it ended") enum32{"passed", "failed", "aborted"}."passed" ("How it ended")] -> w710
                    frame False {
                      # "If Go and Threshold didn't reached, or,\nNo-go and Thres reached, Fail"
                    }
                    frame True {
                      # "If Go and Threshold reached, or,\nNo-go and Thres didn't reach, Pass."
                    }
                  }
                  n193 = local write "Go/No-go LED"(w708) -> ()
                  n194 = call-poly <vilib>:"DAQmx Write.vi"("task/channels in"=w713, "data"=w708, "error in"=w712) -> ("task out"=w714:refnum<k21>, "error out"=w715:errorcluster)  [unwired: 10 in, 1 out]
                  n195 = call <vilib>:"DAQmx Stop Task.vi"("task/channels in"=w714, "error in"=w715) -> ("task out"=w699:refnum<k21>, "error out"=w689:errorcluster)  [unwired: 12 in]
                  n196 = call-poly <vilib>:"DAQmx Write.vi"("task/channels in"=w686, "data"=FALSE, "error in"=w689) -> ("task out"=w685:refnum<k21>, "error out"=w688:errorcluster)  [unwired: 10 in, 1 out]
                  n197 = call <vilib>:"DAQmx Stop Task.vi"("task/channels in"=w685, "error in"=w688) -> ("task out"=w684:refnum<k21>, "error out"=w687:errorcluster)  [unwired: 12 in]
                  n198 = case shown="True" w681 {
                    tunnel: w699 -> [w718 w722]
                    tunnel: [w717 w721] -> w698
                    tunnel: w697 -> [w719 w720]
                    frame True {
                      n199 = Bundle("task out"=w718, "task out"=w719) -> (w717:T5)  [unwired: 1 in]
                    }
                    frame False {
                      n200 = Bundle("task out"=w720, "task out"=w722) -> (w721:T5)  [unwired: 1 in]
                    }
                  }
                }
                frame "init fail" {
                  w847 = FALSE  # No Stop on Init Fail
                }
              }
            }
            frame #2 {
              # "Stop Period"
              n201 = case shown="True" w852 {
                tunnel: [w859 w887] -> w858
                tunnel: w857 -> [w861 w877]
                tunnel: [w861 w884] -> w856
                tunnel: [w860 w862] -> w855
                tunnel: w854 -> [w860 w866]
                tunnel: w853 -> [w859 _]
                frame False {
                }
                frame True {
                  n202 = flat-sequence {
                    tunnel: [w890] -> w883
                    frame #0 {
                      n203 = local read "Stop Duration"() -> (w890:dbl)
                      n204 = local write "Current Period"(u8 3 ("Current Period")) -> ()
                      n205 = local write "Current Thres"(50.0 ("Current Thres 2")) -> ()
                      n206 = property on="Stop Slide" class="Slide (strict)"("Scale.Maximum"=w890, "Maximum"=w890) -> ()  [unwired: 2 in, 2 out]
                    }
                  }
                  n207 = Unbundle(w866) -> ("task out"=w863:refnum<k21>, "task out"=w865:refnum<k21>)
                  n208 = call <vilib>:"DAQmx Start Task.vi"("task/channels in"=w865, "error in"=w877) -> ("task out"=w875:refnum<k21>, "error out"=w876:errorcluster)  [unwired: 12 in]
                  n209 = while {
                    tunnel: [w911] -> w886
                    tunnel: [w892] -> w882
                    tunnel: w883 -> [w908]
                    tunnel: [w907] -> w880
                    tunnel: w876 -> [w905]
                    tunnel: w875 -> [w906]
                    shift-right: [w904] -> w873
                    shift-left: TRUE -> [w902]
                    tunnel: [w891] -> w870
                    i -> [w909]
                    stop <- w894 stop-if-true
                    # "Stop Delay Loop"
                    n210 = Equal To 0?(x=w909) -> (x = 0?=w898:bool)
                    n211 = call "Elapsed Time5"("Time Target (s)"=w908, "Reset"=w898) -> ("Elapsed Time (s)"=w910:dbl, "Time has Elapsed"=w895:bool)  [unwired: 10 in, 6 out]
                    n212 = local read "Buffer Time (s)"() -> (w899:dbl)
                    n213 = local write "Stop Slide"(w910) -> ()
                    n214 = local read "Stop Flash #"() -> (→"Stop Flash # 2":dbl)
                    n215 = local write "Go/No-go LED"(w902) -> ()
                    n216 = local read "Speed"() -> (w892:dbl)
                    n217 = call "Elapsed Time8"("Time Target (s)"=w899, "Reset"=w898) -> ("Time has Elapsed"=w897:bool)  [unwired: 10 in, 7 out]
                    n218 = call-poly <vilib>:"DAQmx Write.vi"("task/channels in"=w906, "data"=w902, "error in"=w905) -> ("task out"=w907:refnum<k21>, "error out"=w911:errorcluster)  [unwired: 10 in, 1 out]
                    n219 = local read "Distance"() -> (w891:dbl)
                    n220 = local read "Stop Stim On (s)"() -> (w893:dbl)
                    n221 = case shown="True" w897 {
                      tunnel: w891 -> [_ w914]
                      tunnel: [FALSE w913] -> w896
                      frame False {
                      }
                      frame True {
                        n222 = local read "Stop Thres."() -> (w915:dbl)
                        n223 = Greater?(x=w915, y=w914) -> (0:w913:bool)
                      }
                    }
                    n224 = call "Elapsed Time7"("Time Target (s)"=w893, "Reset"=w898) -> ("Time has Elapsed"=w903:bool)  [unwired: 10 in, 7 out]
                    n225 = Not And(1:w903, 2:TRUE) -> (0:w904:bool)
                    n226 = Or(x=w896, y=w895) -> (x .or. y?=w894:bool)
                  }
                  n227 = local read "Stop Fail Speed"() -> (w881:dbl)
                  n228 = local read "Stop Thres."() -> (w871:dbl)
                  n229 = And(x=FALSE, y=w873) -> (x .and. y?=w878:bool)
                  n230 = local write "Go/No-go LED"(w878) -> ()
                  n231 = Greater?(x=w881, y=w882) -> (0:→"Stop Speed Reached":bool)
                  n232 = Greater?(x=w871, y=w870) -> (0:w868:bool)
                  n233 = call-poly <vilib>:"DAQmx Write.vi"("task/channels in"=w880, "data"=w878, "error in"=w886) -> ("task out"=w879:refnum<k21>, "error out"=w885:errorcluster)  [unwired: 10 in, 1 out]
                  n234 = Not(x=w868) -> (.not. x?=→"Stop Thres Reached":bool)
                  n235 = call <vilib>:"DAQmx Stop Task.vi"("task/channels in"=w879, "error in"=w885) -> ("task out"=w864:refnum<k21>, "error out"=w884:errorcluster)  [unwired: 12 in]
                  n236 = case "Pass or Fail Stop" shown="False" w868 {
                    tunnel: [pass_fail."Stop Fail" ("How it ended") enum32{"passed", "failed", "aborted"}."passed" ("How it ended")] -> w887
                    frame False {
                    }
                    frame True {
                    }
                  }
                  n237 = Bundle("task out"=w864, "task out"=w863) -> (w862:T5)  [unwired: 1 in]
                }
              }
            }
            frame #3 {
              # "Reward Period"
              n238 = flat-sequence {
                tunnel: [w922] -> w919
                frame #0 {
                  n239 = local read "Conseq. Fails"() -> (w922:i32)
                  n240 = local write "OptoON"(FALSE ("OptoON")) -> ()
                }
              }
              n241 = case shown="0, Default" w920 {
                tunnel: w919 -> [_ w938]
                tunnel: [0 w937] -> w918
                frame 0, Default {
                  # "Only do reward period when it passed"
                  n242 = stacked-sequence {
                    tunnel: [w936] -> w927
                    tunnel: ["Pass Sound"] -> w924
                    frame #0 {
                      n243 = local read "Reward time (s)"() -> (w936:dbl)
                      n244 = local write "Current Period"(4) -> ()
                      n245 = local write "give reward"(TRUE) -> ()
                      n246 = property on="Slide Reward" class="Slide (strict)"("Scale.Maximum"=w936, "Maximum"=w936) -> ()  [unwired: 2 in, 2 out]
                    }
                  }
                  n247 = String To Path(string=w924) -> (path=w926:path)
                  n248 = call <vilib>:"Sound File Read Simple.vi"("path"=w926) -> ("data"=w925:waveform(dbl)[])  [unwired: 7 in, 3 out]
                  n249 = while {
                    tunnel: w927 -> [w932]
                    i -> [w929]
                    stop <- w931 stop-if-true
                    n250 = Equal To 0?(x=w929) -> (x = 0?=w928:bool)
                    n251 = call "Elapsed Time3"("Time Target (s)"=w932, "Reset"=w928) -> ("Elapsed Time (s)"=w930:dbl, "Time has Elapsed"=w931:bool)  [unwired: 10 in, 6 out]
                    n252 = local write "Slide Reward"(w930) -> ()
                  }
                  n253 = call "Play Waveform"("Data"=w925) -> ()  [unwired: 18 in, 1 out]
                }
                frame 1..3 {
                  # "If failed in the last period, skip reward"
                  n254 = String To Path(string="Fail Sound") -> (path=w942:path)
                  n255 = call <vilib>:"Sound File Read Simple.vi"("path"=w942) -> ("data"=w941:waveform(dbl)[])  [unwired: 7 in, 3 out]
                  n256 = Add(x=1, y=w938) -> (x+y=w937:i32)
                  n257 = call "Play Waveform2"("Data"=w941) -> ()  [unwired: 18 in, 1 out]
                }
              }
              n258 = local write "Conseq. Fails"(w918) -> ()
            }
            frame #4 {
              w964 = TRUE ("data")
              # "Inter-trial interval"
              n259 = Get Date/Time In Seconds() -> (seconds since 1Jan1904=w961:timestamp)
              n260 = To Double Precision Float(number=w961) -> (double precision float=w960:dbl)
              n261 = To Double Precision Float(number=w963) -> (double precision float=w962:dbl)
              n262 = local read "NoGo?"() -> (w945:bool)
              n263 = Increment(x=w968) -> (x+1=w947:i32)
              n264 = Boolean To (0,1)(Boolean=w950) -> (0, 1=w949:i16)
              n265 = local write "OptoON"(FALSE ("OptoON")) -> ()
              n266 = local write "Room light"(w964) -> ()
              n267 = local read "Reward Count"() -> (w948:dbl)
              n268 = local write "Slide Trial #"(w947) -> ()
              n269 = call-poly <vilib>:"DAQmx Write.vi"("task/channels in"=w965, "data"=w964, "error in"=w955) -> ("task out"=w954:refnum<k21>, "error out"=w952:errorcluster)  [unwired: 10 in, 1 out]
              n270 = Greater?(x=w967, y=w947) -> (0:w966:bool)
              n271 = Boolean To (0,1)(Boolean=w945) -> (0, 1=w944:i16)
              n272 = Divide(x=w948, y=w947) -> (x/y=w946:dbl)
              n273 = local write "Success %"(w946) -> ()
              n274 = case "Last Trial or not?" shown="True" w966 {
                tunnel: w957 -> [_ w1025]
                tunnel: [_ w1024] -> w958
                tunnel: w954 -> [w1019 w1023]
                tunnel: [w1021 w1023] -> w953
                tunnel: w952 -> [w1017 w1022]
                tunnel: [w1020 w1022] -> w951
                frame False {
                  w1015 = FALSE ("data")
                  # "Last Trial, Do nothing"
                  n275 = local write "Room light"(w1015) -> ()
                  n276 = call-poly <vilib>:"DAQmx Write.vi"("task/channels in"=w1019, "data"=w1015, "error in"=w1017) -> ("task out"=w1018:refnum<k21>, "error out"=w1016:errorcluster)  [unwired: 10 in, 1 out]
                  n277 = call <vilib>:"DAQmx Stop Task.vi"("task/channels in"=w1018, "error in"=w1016) -> ("task out"=w1021:refnum<k21>, "error out"=w1020:errorcluster)  [unwired: 12 in]
                }
                frame True {
                  # "Not the last trial,  inter-trial delay."
                  n278 = stacked-sequence {
                    tunnel: [w1036] -> w1026
                    tunnel: w1025 -> [w1037]
                    tunnel: [w1036] -> w1024
                    frame #0 {
                      n279 = local read "Conseq. Fails"() -> (w1033:i32)
                      n280 = Greater?(x=w1033, y="Fails 2 Penalty") -> (0:w1034:bool)
                      n281 = case shown="True" w1034 {
                        tunnel: ["Fails Penalty (s)" w1045] -> w1040
                        tunnel: ["Fails Penalty (s)" w1044] -> w1039
                        tunnel: w1037 -> [_ w1043]
                        frame True {
                        }
                        frame False {
                          n282 = case shown="1, 2" w1043 {
                            tunnel: [w1047 w1049] -> w1045
                            tunnel: [w1046 w1048] -> w1044
                            frame 0, Default {
                              n283 = local read "Pass Delay Max"() -> (w1047:dbl)
                              n284 = local read "Pass delay Min"() -> (w1046:dbl)
                            }
                            frame 1, 2 {
                              n285 = local read "Fail Delay Max"() -> (w1049:dbl)
                              n286 = local read "Fail Delay Min"() -> (w1048:dbl)
                            }
                          }
                        }
                      }
                      n287 = local write "Current Period"(5) -> ()
                      n288 = Equal?(x=w1040, y=w1039) -> (x = y?=w1041:bool)
                      n289 = case shown="True" w1041 {
                        tunnel: [w1058 w1067] -> w1036
                        tunnel: w1040 -> [w1057 w1067]
                        tunnel: w1039 -> [w1056 _]
                        frame False {
                          # "If min != max; random delay betwen min and max"
                          n290 = Random Number (0-1)() -> (number: 0 to 1=w1065:dbl)
                          n291 = Subtract(x=w1057, y=w1056) -> (x-y=w1066:dbl)
                          n292 = Multiply(x=w1066, y=w1065) -> (x*y=w1064:dbl)
                          n293 = Add(x=w1064, y=w1056) -> (x+y=w1063:dbl)
                          n294 = Multiply(x=w1063, y=1000) -> (x*y=w1060:dbl)
                          n295 = Round To Nearest(number=w1060) -> (nearest integer value=w1059:dbl)
                          n296 = Divide(x=w1059, y=1000) -> (x/y=w1058:dbl)
                        }
                        frame True {
                          # "If min=max; fix delay"
                        }
                      }
                      n297 = case shown="0, Default" w1037 {
                        tunnel: w1036 -> [w1052 w1055]
                        tunnel: [u32 16860 u32 16711680] -> w1038
                        frame 0, Default {
                          n298 = local write "Pass Delay Actual"(w1052) -> ()
                          n299 = local write "Fail Delay Actual"(0.0) -> ()
                        }
                        frame 1 {
                          n300 = local write "Fail Delay Actual"(w1055) -> ()
                          n301 = local write "Pass Delay Actual"(0.0 ("Pass Delay Actual")) -> ()
                        }
                      }
                      n302 = property on="Slide Inter-trail" class="Slide (strict)"("Scale.Maximum"=w1036, "Maximum"=w1036, "Fill Color"=w1038) -> ()  [unwired: 2 in, 2 out]
                    }
                  }
                  n303 = while {
                    tunnel: w1026 -> [w1031]
                    i -> [w1028]
                    stop <- w1030 stop-if-true
                    n304 = Equal To 0?(x=w1028) -> (x = 0?=w1027:bool)
                    n305 = call "Elapsed Time4"("Time Target (s)"=w1031, "Reset"=w1027) -> ("Elapsed Time (s)"=w1029:dbl, "Time has Elapsed"=w1030:bool)  [unwired: 10 in, 6 out]
                    n306 = local write "Slide Inter-trail"(w1029) -> ()
                  }
                }
              }
              n307 = case "Save Trial info" shown="True" w956 {
                tunnel: w947 -> [_ w998]
                tunnel: w962 -> [_ w997]
                tunnel: w960 -> [_ w996]
                tunnel: w959 -> [_ w995]
                tunnel: w958 -> [_ w982]
                tunnel: w957 -> [_ w990]
                tunnel: w949 -> [_ w983]
                tunnel: w944 -> [_ w976]
                frame False {
                }
                frame True {
                  n308 = local read "Init Abort Threshold"() -> (w991:dbl)
                  n309 = local read "Go Duration"() -> (w971:dbl)
                  n310 = local read "Init Delay Actual"() -> (w992:dbl)
                  n311 = local read "NoGo Prob?"() -> (w975:dbl)
                  n312 = local read "Go/noGo Reward Thres"() -> (w974:dbl)
                  n313 = local read "Lick Thr"() -> (w970:dbl)
                  n314 = local read "Fail Repeat Prob"() -> (w977:dbl)
                  n315 = local read "Stim On (s)"() -> (w988:dbl)
                  n316 = local read "Decay"() -> (w978:enum32{"None", "Exp", "Lin", "Log"})
                  n317 = local read "Thr Opto \nRun Factor"() -> (w972:dbl)
                  n318 = case shown="\"None\", Default" w978 {
                    tunnel: [0.0 w1010 w1011 w1012] -> w979
                    frame "None", Default {
                    }
                    frame "Exp" {
                      n319 = local read "Exp rate"() -> (w1010:dbl)
                    }
                    frame "Lin" {
                      n320 = local read "Lin rate"() -> (w1011:dbl)
                    }
                    frame "Log" {
                      n321 = local read "Log rate"() -> (w1012:dbl)
                    }
                  }
                  n322 = local read "Opto Cond"() -> (w973:T1)
                  n323 = local read "Reward time (s)"() -> (w980:dbl)
                  n324 = case shown="0, Default" w990 {
                    tunnel: [w1013 0.0] -> w981
                    frame 0, Default {
                      n325 = local read "Reward Count"() -> (w1013:dbl)
                    }
                    frame 1 {
                    }
                  }
                  n326 = case shown="1" w983 {
                    tunnel: [0.0 w1008] -> w984
                    tunnel: [0.0 w1007] -> w985
                    tunnel: [0.0 w1006] -> w986
                    tunnel: [0.0 w1005] -> w987
                    tunnel: [0.0 w1004] -> w989
                    frame 0, Default {
                    }
                    frame 1 {
                      n327 = local read "Stop Prob"() -> (w1008:dbl)
                      n328 = local read "Stop Delay \nActual (s)"() -> (w1007:dbl)
                      n329 = local read "Stop Duration"() -> (w1006:dbl)
                      n330 = local read "Stop Stim On (s)"() -> (w1004:dbl)
                      n331 = local read "Stop Thres."() -> (w1005:dbl)
                    }
                  }
                  n332 = Build Array(w998, w997, w996, w990, w992, w991, w976, w971, w975, w974, w977, w978, w979, w980, w981, w982, w983, w984, w985, w986, w987, w988, w989, w973, w972, w970) -> (w994:dbl[])
                  n333 = call-poly <vilib>:"Write To Spreadsheet File.vi"("delimiter (\\t)"="," ("delimiter (\\t)"), "append to file? (new file:F)"=TRUE, "1D data"=w994, "file path (dialog if empty)"=w995) -> ()  [unwired: 4 in, 1 out]
                }
              }
            }
            frame #5 {
              # "terminate the trial"
              n334 = local read "Run Trials"() -> (w1068:bool)
            }
          }
        }
        n335 = flat-sequence {
          tunnel: w470 -> [w479]
          tunnel: w469 -> [w482]
          tunnel: w467 -> [w481]
          tunnel: w459 -> [w474]
          frame #0 {
            n336 = Unbundle(w479) -> ("task out"=w478:refnum<k21>, "task out"=w477:refnum<k21>)
            n337 = call <vilib>:"DAQmx Clear Task.vi"("task in"=w482, "error in"=w481) -> ("error out"=w476:errorcluster)  [unwired: 13 in]
            n338 = local write "Run Trials"(FALSE ("Run Trials")) -> ()
            n339 = call <vilib>:"DAQmx Clear Task.vi"("task in"=w474) -> ()  [unwired: 14 in, 1 out]
            n340 = call <vilib>:"DAQmx Clear Task.vi"("task in"=w477, "error in"=w476) -> ("error out"=w475:errorcluster)  [unwired: 13 in]
            n341 = call <vilib>:"DAQmx Clear Task.vi"("task in"=w478, "error in"=w475) -> ()  [unwired: 13 in, 1 out]
          }
        }
      }
    }
    n342 = local read "Wheel Test"() -> (w18:bool)
    n343 = And(x=w7, y=w5) -> (x .and. y?=w6:bool)
    n344 = Or(x=w5, y=w18) -> (x .or. y?=w3:bool)
    n345 = Compound Arithmetic op=OR(w5, "Shutter Click") -> (w4:bool)
    n346 = case shown="True" w3 {
      tunnel: w5 -> [_ w151]
      tunnel: w6 -> [_ w141]
      frame False {
      }
      frame True {
        w125 = 10083 items=["default"=-1, "RSE"=10083, "NRSE"=10078, "Differential"=10106, "Pseudodifferential"=12529] ("input terminal configuration")
        n347 = flat-sequence {
          tunnel: [w329] -> w148
          tunnel: [w328] -> w147
          tunnel: [w327] -> w123
          frame #0 {
            w325 = 0.0
            w327 = u32 1073684535 items=["Null"=0, "USB Interrupt"=1073684535]
            n348 = VISA Open(VISA resource name="Wheel Monitor Channel") -> (VISA resource name=w333:refnum<visa-resource-name>, error out=w332:errorcluster)  [unwired: 1 in, 3 out]
            n349 = VISA Enable Event(8:w332, 10:w327, 11:w333) -> (0:w326:errorcluster, 3:w331:refnum<visa-resource-name>)  [unwired: 1 out]
            n350 = while {
              tunnel: w331 -> [w342]
              tunnel: [w341] -> w330
              tunnel: w327 -> [w335]
              stop <- w336 stop-if-true
              n351 = VISA Wait on Event(7:1, 10:w335, 11:w342) -> (1:w343:refnum<visa-resource-name>, 3:w341:refnum<visa-resource-name>)  [unwired: 1 in, 3 out]
              n352 = call <vilib>:"VISA Get USB Interrupt Data.vi"("VISA USB Intr Event"=w343) -> ("data buffer"=w338:u8[], "VISA USB Intr Event out"=w340:refnum<visa-resource-name>)  [unwired: 1 in, 8 out]
              n353 = Add Array Elements(numeric array=w338) -> (sum=w337:u8)
              n354 = Equal To 0?(x=w337) -> (x = 0?=w336:bool)
              n355 = VISA Close(VISA resource name=w340) -> ()  [unwired: 1 in, 1 out]
            }
            n356 = local write "Speed"(w325) -> ()
            n357 = VISA Discard Events(8:w326, 11:w330) -> (0:w328:errorcluster, 3:w329:refnum<visa-resource-name>)  [unwired: 2 in]
            "Distance" <- w325
          }
        }
        n358 = local read "Analog Lick Chan"() -> (w126:tag)
        n359 = call-poly <vilib>:"DAQmx Create Virtual Channel.vi"("input terminal configuration"=w125, "physical channels"=w126) -> ("task out"=w124:refnum<k21>)  [unwired: 12 in, 1 out]
        n360 = local read "Digital In Channel"() -> (w140:tag)
        n361 = call-poly <vilib>:"DAQmx Create Virtual Channel.vi"("lines"=w140) -> ("task out"=w139:refnum<k21>)  [unwired: 13 in, 1 out]
        n362 = Obtain Queue(name (unnamed)="DataQueue", element data type="Queue") -> (queue out=w145:refnum<queue>, error out=w144:errorcluster)  [unwired: 3 in, 1 out]
        n363 = while {
          tunnel: [w208] -> w152
          tunnel: w145 -> [w206]
          tunnel: w144 -> [w205]
          tunnel: w139 -> [w204]
          tunnel: [w203] -> w138
          tunnel: [w202] -> w137
          tunnel: w124 -> [w201]
          shift-right: [w175] -> _
          shift-left: "Queue" -> [w207]
          tunnel: [w174] -> w121
          stop <- w178 continue-if-true
          n364 = flat-sequence {
            tunnel: w204 -> [w250]
            tunnel: [w249] -> w202
            tunnel: w201 -> [w248]
            tunnel: [w247] -> w199
            tunnel: [w246] -> w193
            tunnel: [w245] -> w182
            tunnel: [w244] -> w172
            tunnel: [w243] -> w171
            tunnel: [w242] -> w174
            frame #0 {
              n365 = Get Date/Time In Seconds() -> (seconds since 1Jan1904=w247:timestamp)
              n366 = local read "Speed"() -> (w244:dbl)
              n367 = call-poly <vilib>:"DAQmx Read.vi"("task/channels in"=w248) -> ("task out"=w242:refnum<k21>, "data"=w245:dbl)  [unwired: 12 in, 1 out]
              n368 = local read "Distance"() -> (w243:dbl)
              n369 = call-poly <vilib>:"DAQmx Read.vi"("task/channels in"=w250) -> ("task out"=w249:refnum<k21>, "data"=w246:bool)  [unwired: 12 in, 1 out]
            }
          }
          n370 = local read "Sample Time Interval (ms)"() -> (w164:u32)
          n371 = Greater?(x=w171, y=0.0) -> (0:w169:bool)
          n372 = local read "Current Thres"() -> (w165:dbl)
          n373 = Boolean To (0,1)(Boolean=w169) -> (0, 1=w168:i16)
          n374 = Multiply(x=w168, y="Decay") -> (x*y=w166:u32)
          n375 = case shown="3" w166 {
            tunnel: w171 -> [w223 w231 w240 w241]
            tunnel: [w222 w232 w238 w241] -> w163
            tunnel: w165 -> [_ w229 w233 _]
            tunnel: w164 -> [_ w227 _ _]
            frame 1 {
              # "Exp"
              n376 = Subtract(x=1, y="Exp rate") -> (x-y=w221:dbl)
              n377 = Multiply(x=w223, y=w221) -> (x*y=w222:dbl)
            }
            frame 2 {
              # "linear"
              n378 = Multiply(x="Lin rate", y=w229) -> (x*y=w226:dbl)
              n379 = Multiply(x=w226, y=w227) -> (x*y=w228:dbl)
              n380 = Divide(x=w228, y=1000) -> (x/y=w225:dbl)
              n381 = Subtract(x=w231, y=w225) -> (x-y=w232:dbl)
            }
            frame 3 {
              # "log"
              n382 = local read "Log rate"() -> (w234:dbl)
              n383 = Add(x=1, y=w234) -> (x+y=w236:dbl)
              n384 = Subtract(x=w233, y=w240) -> (x-y=w239:dbl)
              n385 = Multiply(x=w239, y=w236) -> (x*y=w237:dbl)
              n386 = Subtract(x=w233, y=w237) -> (x-y=w238:dbl)
            }
            frame 0, Default {
            }
          }
          n387 = local read "reset distance"() -> (w161:bool)
          n388 = Less Than 0?(x=w163) -> (x < 0?=w162:bool)
          n389 = Or(x=w162, y=w161) -> (x .or. y?=w160:bool)
          n390 = case shown="True" w160 {
            tunnel: [w209 0.0] -> w159
            tunnel: w163 -> [w209 _]
            frame False {
            }
            frame True {
              "reset distance" <- FALSE
            }
          }
          n391 = local write "Distance"(w159) -> ()
          n392 = local read "OptoON"() -> (w191:bool)
          n393 = Multiply(x="Scale", y=w182) -> (x*y=w186:dbl)
          n394 = Add(x="x", y=w186) -> (x+y=w184:dbl)
          "x*y" <- w184
          n395 = Divide(x=w159, y=w165) -> (x/y=w179:dbl)
          n396 = Greater?(x=w182, y="Lick Thr") -> (0:w181:bool)
          "Ana Lick?" <- w181
          n397 = local write "In"(w193) -> ()
          n398 = Boolean To (0,1)(Boolean=w193) -> (0, 1=w192:i16)
          n399 = Divide(x="Current Period", y=10) -> (x/y=w194:dbl)
          n400 = Boolean To (0,1)(Boolean=w191) -> (0, 1=w190:i16)
          n401 = To Double Precision Float(number=w199) -> (double precision float=w198:dbl)
          n402 = Add(x="Current Trial", y=w194) -> (x+y=w173:dbl)
          n403 = Divide(x=w190, y=i16 2) -> (x/y=w188:dbl)
          n404 = Boolean To (0,1)(Boolean=w181) -> (0, 1=w180:i16)
          n405 = Bundle By Name(cluster=w207, "Trial"=w173, "Speed"=w172, "Distance"=w159, "Time"=w198, "Dig In 1"=w192, "Opto"=w190, "Ana Lick"=w182, "Trial"=w180) -> (w175:T2)
          n406 = Bundle("Speed"=w172, w179, w192, w188, w184) -> (w200:cluster{"Speed":dbl, dbl, i16, dbl, dbl})  [unwired: 1 in]
          n407 = flat-sequence {
            tunnel: [w218] -> w208
            tunnel: w206 -> [w217]
            tunnel: w205 -> [w216]
            tunnel: [w215] -> w203
            tunnel: w200 -> [w214]
            tunnel: w175 -> [w213]
            tunnel: w164 -> [w212]
            frame #0 {
              n408 = Enqueue Element(queue=w217, element=w213, error in (no error)=w216) -> (queue out=w218:refnum<queue>, error out=w215:errorcluster)  [unwired: 1 in, 1 out]
              n409 = Wait Until Next ms Multiple(millisecond multiple=w212) -> ()  [unwired: 1 out]
              "Wheel Graph" <- w214
            }
          }
          n410 = local read "Wheel Test"() -> (w177:bool)
          n411 = local read "Run Trials"() -> (w176:bool)
          n412 = Or(x=w177, y=w176) -> (x .or. y?=w178:bool)
        }
        n413 = while {
          tunnel: w151 -> [_]
          tunnel: [w268] -> w150
          tunnel: [w267] -> w149
          tunnel: w148 -> [w266]
          tunnel: w147 -> [w265]
          tunnel: w123 -> [w256]
          shift-right: [w251] -> _
          shift-left: 1000 ("timeout (0)") -> [w264]
          stop <- w259 continue-if-true
          n414 = VISA Wait on Event(7:w264, 8:w265, 10:w256, 11:w266) -> (0:w253:errorcluster, 1:w255:refnum<visa-resource-name>, 2:w257:u32, 3:w261:refnum<visa-resource-name>)  [unwired: 1 out]
          n415 = Equal?(x=w256, y=w257) -> (x = y?=w258:bool)
          n416 = case shown="True" w258 {
            tunnel: w255 -> [w272 w282]
            tunnel: [w272 w281] -> w254
            tunnel: w253 -> [w271 w280]
            tunnel: [w271 w279] -> w252
            tunnel: [1000 1] -> w251
            frame False {
              # "Time out. No input from the mouse. Need to set the speed to 0 immediately"
              n417 = local write "Speed"(0.0) -> ()
            }
            frame True {
              w300 = 127
              # "threshold"
              # "no negative"
              # "decay"
              # "z"
              # "y"
              # "USB interrupt. Only run when mouse is moving"
              n418 = call <vilib>:"VISA Get USB Interrupt Data.vi"("error in (no error)"=w280, "VISA USB Intr Event"=w282) -> ("error out"=w279:errorcluster, "data buffer"=w278:u8[], "VISA USB Intr Event out"=w281:refnum<visa-resource-name>)  [unwired: 7 out]
              n419 = Index Array(array=w278, index=2) -> (element=w292:u8)
              n420 = Index Array(array=w278, index=4) -> (element=w291:u8)
              n421 = Greater?(x=w292, y=w300) -> (0:w307:bool)
              n422 = Greater?(x=w291, y=w300) -> (0:w308:bool)
              n423 = case shown="True" w307 {
                tunnel: w292 -> [w317 w319]
                tunnel: [w317 w318] -> w304
                frame False {
                }
                frame True {
                  n424 = Subtract(x=w319, y=256) -> (x-y=w318:i32)
                }
              }
              n425 = case shown="True" w308 {
                tunnel: w291 -> [w321 w323]
                tunnel: [w321 w322] -> w305
                frame False {
                }
                frame True {
                  n426 = Subtract(x=w323, y=256) -> (x-y=w322:i32)
                }
              }
              n427 = Divide(x=w304, y=w300) -> (x/y=w290:dbl)
              n428 = Divide(x=w305, y=w300) -> (x/y=w298:dbl)
              n429 = case shown="False" "Wheel direction" {
                tunnel: [1 -1] -> w289
                frame False {
                }
                frame True {
                }
              }
              n430 = Square(x=w290) -> (x^2=w297:dbl)
              n431 = Square(x=w298) -> (x^2=w296:dbl)
              n432 = Add(x=w297, y=w296) -> (x+y=w306:dbl)
              n433 = Multiply(x=w289, y=w290) -> (x*y=w303:dbl)
              n434 = Square Root(x=w306) -> (sqrt(x)=w295:dbl)
              n435 = Sign(1:w303) -> (0:w294:dbl)
              n436 = Multiply(x=w294, y=w295) -> (x*y=w293:dbl)
              n437 = local read "Distance"() -> (w288:dbl)
              n438 = local write "Speed"(w293) -> ()
              n439 = Add(x=w293, y=w288) -> (x+y=w274:dbl)
              n440 = local read "Thr Opto \nRun Factor"() -> (w275:dbl)
              n441 = Less Than 0?(x=w274) -> (x < 0?=w287:bool)
              n442 = local read "Current Thres"() -> (w276:dbl)
              n443 = case shown="True" w287 {
                tunnel: [w310 0.0] -> w284
                tunnel: w274 -> [w310 _]
                frame False {
                }
                frame True {
                }
              }
              n444 = Multiply(x=w276, y=w275) -> (x*y=w286:dbl)
              n445 = Greater Or Equal?(x=w284, y=w276) -> (x >= y?=w273:bool)
              n446 = Greater Or Equal?(x=w284, y=w286) -> (x >= y?=w285:bool)
              n447 = case shown="True" w273 {
                tunnel: [w312 0.0] -> w283
                tunnel: w284 -> [w312 _]
                frame False {
                }
                frame True {
                  n448 = local write "Thres reached"(TRUE) -> ()
                }
              }
              n449 = case shown="True" w285 {
                frame False {
                }
                frame True {
                  n450 = local write "Opto RUN Thr"(TRUE ("Opto RUN Thr")) -> ()
                }
              }
              n451 = local write "Distance"(w283) -> ()
            }
          }
          n452 = VISA Close(VISA resource name=w254, error in (no error)=w252) -> (error out=w260:errorcluster)
          n453 = VISA Discard Events(8:w260, 11:w261) -> (0:w267:errorcluster, 3:w268:refnum<visa-resource-name>)  [unwired: 2 in]
          n454 = local read "Wheel Test"() -> (w263:bool)
          n455 = local read "Run Trials"() -> (w262:bool)
          n456 = Or(x=w263, y=w262) -> (x .or. y?=w259:bool)
        }
        n457 = case shown="True" w141 {
          tunnel: [refnum<file> refnum ("refnum out") w397] -> w154
          tunnel: [errorcluster {"status"=FALSE, "code"=0, "source"=""} ("error out") w396] -> w155
          frame False {
          }
          frame True {
            n458 = local read "Data File Location"() -> (w395:path)
            n459 = Open/Create/Replace File(file path (use dialog)=w395, operation (0:open)=T3."open or create") -> (refnum out=w394:refnum<file>, error out=w382:errorcluster)  [unwired: 4 in, 1 out]
            n460 = Build Array("Trial", "Speed", "Distance", "Time", "Dig In 1", "Opto" ("element"), "Ana Lick" ("element"), "AnaDig Lick" ("element")) -> (w399:string[])
            n461 = Set File Position(offset (in bytes) (0)=0, refnum=w394, from (0:start)=1, error in=w382) -> (refnum out=w393:refnum<file>, error out=w381:errorcluster)
            n462 = Array To Spreadsheet String(delimiter (Tab)=",", array=w399, 3:"%s") -> (spreadsheet string=w400:string)
            n463 = Write to Text File(file (use dialog)=w393, text=w400, error in=w381) -> (refnum out=w397:refnum<file>, error out=w396:errorcluster)  [unwired: 1 in, 1 out]
          }
        }
        n464 = local read "No-Go/Stop Channel"() -> (w134:tag)
        n465 = while {
          tunnel: w145 -> [w415]
          tunnel: w144 -> [w414]
          tunnel: w154 -> [w412]
          tunnel: w155 -> [w411]
          tunnel: [w410] -> w156
          tunnel: [w409] -> w157
          stop <- w407 continue-if-true
          n466 = local read "Save"() -> (w404:bool)
          n467 = Dequeue Element(queue=w415, error in (no error)=w414) -> (element=w413:T2, timed out?=w402:bool)  [unwired: 1 in, 2 out]
          n468 = Not(x=w402) -> (.not. x?=w403:bool)
          n469 = And(x=w403, y=w404) -> (x .and. y?=w405:bool)
          n470 = case shown="True" w405 {
            tunnel: w413 -> [_ w419]
            tunnel: w412 -> [w417 w426]
            tunnel: w411 -> [w416 w425]
            tunnel: [w417 w424] -> w410
            tunnel: [w416 w423] -> w409
            frame False {
            }
            frame True {
              n471 = Cluster To Array(cluster=w419) -> (array=w418:dbl[])
              n472 = Array To Spreadsheet String(delimiter (Tab)=",", array=w418, 3:"%0.3f" ("format string")) -> (spreadsheet string=w421:string)
              n473 = Write to Text File(file (use dialog)=w426, text=w421, error in=w425) -> (refnum out=w424:refnum<file>, error out=w423:errorcluster)  [unwired: 1 in, 1 out]
            }
          }
          n474 = local read "Wheel Test"() -> (w406:bool)
          n475 = local read "Run Trials"() -> (w408:bool)
          n476 = Or(x=w406, y=w408) -> (x .or. y?=w407:bool)
        }
        n477 = call-poly <vilib>:"DAQmx Create Virtual Channel.vi"("lines"=w134) -> ("task out"=w132:refnum<k21>, "error out"=w129:errorcluster)  [unwired: 13 in]
        n478 = local read "control puff"() -> (w133:bool)
        n479 = case shown="True" w133 {
          tunnel: w132 -> [w346 w352]
          tunnel: [w346 w351] -> w131
          tunnel: w129 -> [w345 w349]
          tunnel: [w345 w348] -> w128
          tunnel: [FALSE w347] -> w127
          frame False {
          }
          frame True {
            n480 = while {
              tunnel: w352 -> [w366]
              tunnel: [w365] -> w351
              shift-right: [w363] -> _
              shift-left: TRUE -> [w357]
              tunnel: [FALSE] -> w347
              tunnel: w349 -> [w355]
              tunnel: [w354] -> w348
              stop <- w360 continue-if-true
              n481 = flat-sequence {
                tunnel: w366 -> [w371]
                tunnel: [w370] -> w364
                tunnel: [w367] -> w358
                tunnel: w357 -> [w367]
                tunnel: w355 -> [w369]
                tunnel: [w368] -> w353
                tunnel: [w374] -> w365
                tunnel: w364 -> [w374]
                tunnel: [w373] -> w359
                tunnel: w358 -> [w373]
                tunnel: [w372] -> w354
                tunnel: w353 -> [w372]
                frame #0 {
                  n482 = call-poly <vilib>:"DAQmx Write.vi"("task/channels in"=w371, "data"=w367, "error in"=w369) -> ("task out"=w370:refnum<k21>, "error out"=w368:errorcluster)  [unwired: 10 in, 1 out]
                }
                frame #1 {
                  n483 = Multiply(x="control puff interval", y=1000.0) -> (x*y=w375:dbl)
                  n484 = Wait (ms)(milliseconds to wait=w375) -> ()  [unwired: 1 out]
                }
              }
              n485 = local read "Wheel Test"() -> (w362:bool)
              n486 = local read "Run Trials"() -> (w361:bool)
              n487 = Or(x=w362, y=w361) -> (x .or. y?=w360:bool)
              n488 = Not(x=w359) -> (.not. x?=w363:bool)
            }
          }
        }
        n489 = Close File(refnum=w156, error in=w157) -> ()  [unwired: 2 out]
        n490 = call-poly <vilib>:"DAQmx Write.vi"("task/channels in"=w131, "auto start"=TRUE, "data"=w127, "error in"=w128) -> ("task out"=w130:refnum<k21>, "error out"=w136:errorcluster)  [unwired: 9 in, 1 out]
        n491 = call <vilib>:"DAQmx Clear Task.vi"("task in"=w130, "error in"=w136) -> ()  [unwired: 13 in, 1 out]
        n492 = call <vilib>:"DAQmx Stop Task.vi"("task/channels in"=w121) -> ("task out"=w118:refnum<k21>, "error out"=w117:errorcluster)  [unwired: 13 in]
        n493 = call <vilib>:"DAQmx Stop Task.vi"("task/channels in"=w137) -> ("task out"=w120:refnum<k21>, "error out"=w119:errorcluster)  [unwired: 13 in]
        n494 = VISA Close(VISA resource name=w150, error in (no error)=w149) -> (error out=w142:errorcluster)
        n495 = call <vilib>:"DAQmx Clear Task.vi"("task in"=w118, "error in"=w117) -> ()  [unwired: 13 in, 1 out]
        n496 = call <vilib>:"DAQmx Clear Task.vi"("task in"=w120, "error in"=w119) -> ()  [unwired: 13 in, 1 out]
        n497 = Release Queue(queue=w152, force destroy? (F)=TRUE, error in (no error)=w138) -> (error out=w143:errorcluster)  [unwired: 2 out]
        n498 = Merge Errors(w143, w142) -> ()  [unwired: 1 out]
      }
    }
    n499 = case shown="True" w4 {
      tunnel: "Shutter Click" -> [_ w61]
      frame False {
      }
      frame True {
        n500 = call-poly <vilib>:"DAQmx Create Virtual Channel.vi"("lines"="Shutter Channel") -> ("task out"=w63:refnum<k21>, "error out"=w64:errorcluster)  [unwired: 13 in]
        n501 = call <vilib>:"DAQmx Start Task.vi"("task/channels in"=w63, "error in"=w64) -> ("task out"=w65:refnum<k21>, "error out"=w66:errorcluster)  [unwired: 12 in]
        n502 = while "Shutter Control Loop" {
          tunnel: w65 -> [w82]
          tunnel: w66 -> [w81]
          tunnel: [w80] -> w72
          tunnel: [w79] -> w73
          shift-right: [w83] -> _
          shift-left: 0.0 -> [w84]
          tunnel: w61 -> [w76]
          stop <- w78 continue-if-true
          n503 = local read "give reward"() -> (w75:bool)
          n504 = Or(x=w76, y=w75) -> (x .or. y?=w77:bool)
          n505 = case shown="True" w77 {
            tunnel: w84 -> [w87 w98]
            tunnel: [w87 w97] -> w83
            tunnel: w75 -> [_ w96]
            tunnel: w82 -> [w86 w95]
            tunnel: w81 -> [w85 w94]
            tunnel: [w86 w89] -> w80
            tunnel: [w85 w88] -> w79
            frame False {
            }
            frame True {
              n506 = flat-sequence {
                tunnel: w95 -> [w103]
                tunnel: w94 -> [w102]
                tunnel: [w101] -> w92
                tunnel: [w100] -> w90
                tunnel: [w107] -> w93
                tunnel: w92 -> [w107]
                tunnel: [w106] -> w91
                tunnel: w90 -> [w106]
                tunnel: w93 -> [w113]
                tunnel: w91 -> [w112]
                tunnel: [w111] -> w89
                tunnel: [w110] -> w88
                frame #0 {
                  w99 = TRUE
                  n507 = local write "Shutter"(w99) -> ()
                  n508 = call-poly <vilib>:"DAQmx Write.vi"("task/channels in"=w103, "data"=w99, "error in"=w102) -> ("task out"=w101:refnum<k21>, "error out"=w100:errorcluster)  [unwired: 10 in, 1 out]
                }
                frame #1 {
                  n509 = local read "Shutter Duration"() -> (w108:dbl)
                  n510 = Multiply(x=1000, y=w108) -> (x*y=w105:dbl)
                  n511 = Wait (ms)(milliseconds to wait=w105) -> ()  [unwired: 1 out]
                }
                frame #2 {
                  w109 = FALSE ("data")
                  n512 = local write "give reward"(w109) -> ()
                  n513 = call-poly <vilib>:"DAQmx Write.vi"("task/channels in"=w113, "data"=w109, "error in"=w112) -> ("task out"=w111:refnum<k21>, "error out"=w110:errorcluster)  [unwired: 10 in, 1 out]
                  n514 = local write "Shutter"(w109) -> ()
                }
              }
              n515 = case shown="True" w96 {
                tunnel: w98 -> [w114 w116]
                tunnel: [w114 w115] -> w97
                frame False {
                }
                frame True {
                  n516 = Increment(x=w116) -> (x+1=w115:dbl)
                }
              }
            }
          }
          "Reward Count" <- w83
          n517 = local read "Run Trials"() -> (w78:bool)
        }
        n518 = call-poly <vilib>:"DAQmx Write.vi"("task/channels in"=w72, "data"=FALSE, "error in"=w73) -> ("task out"=w69:refnum<k21>, "error out"=w70:errorcluster)  [unwired: 10 in, 1 out]
        n519 = call <vilib>:"DAQmx Stop Task.vi"("task/channels in"=w69, "error in"=w70) -> ("task out"=w67:refnum<k21>, "error out"=w68:errorcluster)  [unwired: 12 in]
        n520 = call <vilib>:"DAQmx Clear Task.vi"("task in"=w67, "error in"=w68) -> ()  [unwired: 13 in, 1 out]
      }
    }
    n521 = local read "Flash test"() -> (w9:bool)
    n522 = Not(x=w5) -> (.not. x?=w12:bool)
    n523 = Not(x=w5) -> (.not. x?=w11:bool)
    n524 = And(x=w9, y=w11) -> (x .and. y?=w10:bool)
    n525 = Or(x="Pass sound play", y="Fail sound play") -> (x .or. y?=w13:bool)
    n526 = case "Go/No-go LED Test" shown="True" w10 {
      frame False {
      }
      frame True {
        n527 = local read "Go Channel"() -> (w30:tag)
        n528 = call-poly <vilib>:"DAQmx Create Virtual Channel.vi"("lines"=w30) -> ("task out"=w28:refnum<k21>, "error out"=w27:errorcluster)  [unwired: 13 in]
        n529 = while {
          tunnel: [w41] -> w29
          tunnel: [w40] -> w24
          tunnel: w28 -> [w39]
          tunnel: w27 -> [w38]
          shift-right: [w33] -> _
          shift-left: TRUE -> [w37]
          tunnel: [FALSE] -> w21
          stop <- w32 continue-if-true
          n530 = flat-sequence {
            tunnel: w39 -> [w44]
            tunnel: w38 -> [w43]
            tunnel: w37 -> [w42]
            tunnel: [w46] -> w36
            tunnel: [w45] -> w35
            tunnel: [w42] -> w34
            tunnel: [w53] -> w40
            tunnel: [w54] -> w41
            tunnel: w36 -> [w54]
            tunnel: w35 -> [w53]
            tunnel: [w51] -> w33
            tunnel: w34 -> [w52]
            frame #0 {
              n531 = local write "Go/No-go LED"(w42) -> ()
              n532 = call-poly <vilib>:"DAQmx Write.vi"("task/channels in"=w44, "auto start"=TRUE, "data"=w42, "error in"=w43) -> ("task out"=w46:refnum<k21>, "error out"=w45:errorcluster)  [unwired: 9 in, 1 out]
            }
            frame #1 {
              n533 = local read "Flashing Interval"() -> (w49:dbl)
              n534 = Not(x=w52) -> (.not. x?=w51:bool)
              n535 = Multiply(x=w49, y=1000.0) -> (x*y=w50:dbl)
              n536 = Wait (ms)(milliseconds to wait=w50) -> ()  [unwired: 1 out]
            }
          }
          n537 = local read "Flash test"() -> (w32:bool)
        }
        n538 = local write "Go/No-go LED"(w21) -> ()
        n539 = call-poly <vilib>:"DAQmx Write.vi"("task/channels in"=w29, "auto start"=TRUE, "data"=w21, "error in"=w24) -> ("task out"=w25:refnum<k21>, "error out"=w23:errorcluster)  [unwired: 9 in, 1 out]
        n540 = call <vilib>:"DAQmx Clear Task.vi"("task in"=w25, "error in"=w23) -> ()  [unwired: 13 in, 1 out]
      }
    }
    n541 = event shown="[1] \"Sample Rate (Hz)\": Value Change" {
      selector: _ -> [_ _ _ _ _]
      dyn-events: _ -> [_ _ _ _ _]
      timeout: 1 -> [_ _ _ _ _]
      event "Room light test": Value Change {
        n542 = event-data() -> ("NewVal"=w427:bool)  [unwired: 1 in, 5 out]
        n543 = local read "Room Light Channel"() -> (w433:tag)
        n544 = call-poly <vilib>:"DAQmx Create Virtual Channel.vi"("lines"=w433) -> ("task out"=w432:refnum<k21>, "error out"=w431:errorcluster)  [unwired: 13 in]
        n545 = call-poly <vilib>:"DAQmx Write.vi"("task/channels in"=w432, "auto start"=TRUE, "data"=w427, "error in"=w431) -> ("task out"=w429:refnum<k21>, "error out"=w428:errorcluster)  [unwired: 9 in, 1 out]
        n546 = local write "Room light"(w427) -> ()
        n547 = call <vilib>:"DAQmx Clear Task.vi"("task in"=w429, "error in"=w428) -> ()  [unwired: 13 in, 1 out]
      }
      event "Sample Rate (Hz)": Value Change {
        n548 = event-data() -> ("NewVal"=w437:u32)  [unwired: 1 in, 5 out]
        n549 = Divide(x=1000, y=w437) -> (x/y=w435:dbl)
        n550 = Round To Nearest(number=w435) -> (nearest integer value=w434:dbl)
        n551 = local write "Sample Time Interval (ms)"(w434) -> ()
      }
      event "Data File Location": Value Change {
        w439 = ".csv"
        n552 = event-data() -> ("NewVal"=w444:path)  [unwired: 1 in, 5 out]
        n553 = Strip Path(path=w444) -> (stripped path=w438:path, name=w440:string)
        n554 = String Length(string=w440) -> (length=w446:i32)
        n555 = Subtract(x=w446, y=4) -> (x-y=w443:i32)
        n556 = String Subset(string=w440, offset (0)=w443) -> (substring=w442:string)  [unwired: 1 in]
        n557 = Not Equal?(x=w442, y=w439) -> (x != y?=w441:bool)
        n558 = case shown="True" w441 {
          tunnel: w440 -> [_ w451]
          tunnel: w439 -> [_ w450]
          tunnel: w438 -> [_ w448]
          frame False {
          }
          frame True {
            n559 = Concatenate Strings(w451, w450) -> (w449:string)
            n560 = Build Path(base path=w448, name or relative path=w449) -> (appended path=w447:path)
            n561 = local write "Data File Location"(w447) -> ()
          }
        }
      }
      event "Solid test": Value Change {
        n562 = event-data() -> ("NewVal"=w452:bool)  [unwired: 1 in, 5 out]
        n563 = local read "Go Channel"() -> (w458:tag)
        n564 = call-poly <vilib>:"DAQmx Create Virtual Channel.vi"("lines"=w458) -> ("task out"=w457:refnum<k21>, "error out"=w456:errorcluster)  [unwired: 13 in]
        n565 = local write "Go/No-go LED"(w452) -> ()
        n566 = call-poly <vilib>:"DAQmx Write.vi"("task/channels in"=w457, "auto start"=TRUE, "data"=w452, "error in"=w456) -> ("task out"=w454:refnum<k21>, "error out"=w453:errorcluster)  [unwired: 9 in, 1 out]
        n567 = call <vilib>:"DAQmx Clear Task.vi"("task in"=w454, "error in"=w453) -> ()  [unwired: 13 in, 1 out]
      }
      event Timeout {
        n568 = event-data() -> ()  [unwired: 1 in, 3 out]
      }
    }
    n569 = And(x=w13, y=w12) -> (x .and. y?=w15:bool)
    n570 = case "Sound test" shown="False" w15 {
      tunnel: "Pass sound play" -> [_ w58]
      frame False {
      }
      frame True {
        n571 = case shown="False" w58 {
          tunnel: [w59 w60] -> w55
          frame False {
            n572 = local read "Fail Sound"() -> (w59:string)
          }
          frame True {
            n573 = local read "Pass Sound"() -> (w60:string)
          }
        }
        n574 = String To Path(string=w55) -> (path=w57:path)
        n575 = call <vilib>:"Sound File Read Simple.vi"("path"=w57) -> ("data"=w56:waveform(dbl)[])  [unwired: 7 in, 3 out]
        n576 = call "Play Waveform3"("Data"=w56) -> ()  [unwired: 18 in, 1 out]
      }
    }
    n577 = local read "exit"() -> (w20:bool)
  }
